vi "Certi Recall.vi"(4 "Value":string[][](array[string]), 5 "큐 입력":refnum<queue>, 6 "NumRows":u32, 7 "입력 클러스터":T1, 8 "에러 입력":errorcluster caption="에러 입력(에러 없음)", 10 "Text in":string, 11 "Func_ext in":string) -> (0 "에러 출력":errorcluster, 3 "Func_ext Out":string)   [LabVIEW 2020]
uses:
  Controls/Clst_Initialize Input.ctl
  Controls/Cmd_Var Data IO.ctl
  Variables/Global_Cal Info.vi
  Public/Polymorph/Table Initialize_Str.vi
  Public/Polymorph/Table Initialize_2D.vi
  Public/Polymorph/Rmv Empt Arr_2D Str.vi
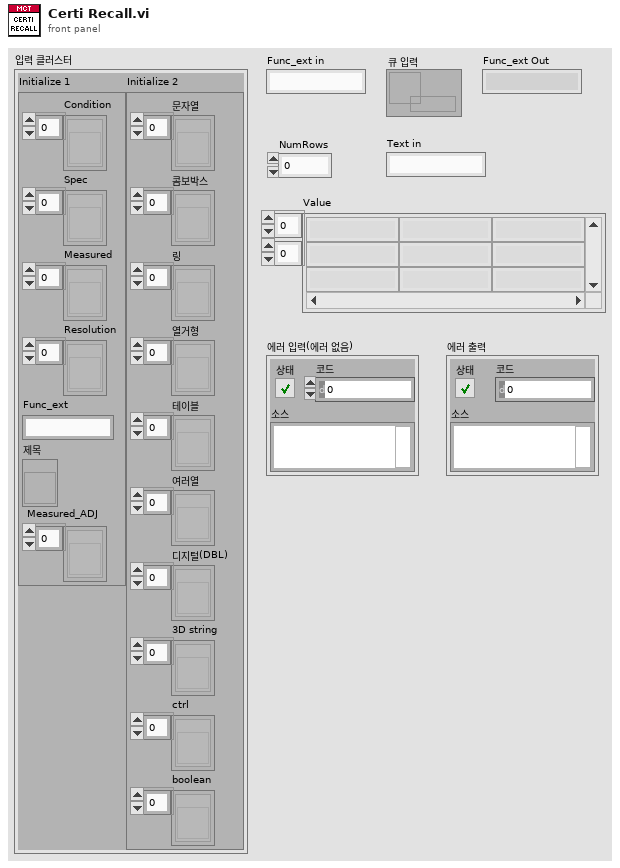
[diagram p1: front panel]
types:
  T1 = typedef "Clst_Initialize Input.ctl" = cluster{"Initialize 1":cluster{"Condition":refnum<vi>[], "Spec":refnum<vi>[], "Measured":refnum<vi>[], "Resolution":refnum<vi>[], "Func_ext":string, "제목":refnum<vi>, "Measured_ADJ":refnum<vi>[]}, "Initialize 2":cluster{"문자열":refnum<vi>[], "콤보박스":refnum<vi>[], "링":refnum<vi>[], "열거형":refnum<vi>[], "테이블":refnum<vi>[], "여러열":refnum<vi>[], "디지털(DBL)":refnum<vi>[], "3D string":refnum<vi>[], "ctrl":refnum<vi>[], "boolean":refnum<vi>[]}}
  T2 = cluster{"세부분류코드":string, "형식":string, "옵션":string, "측정기명":string, "EXCEL파일명":string, "TEMP":string}
  T3 = typedef "Cmd_Var Data IO.ctl" = enum16{"Condition", "Condition Default", "Condition_Temp", "Resolution", "Resolution Default", "Resolution Old", "Spec", "Spec Default", "Spec Old", "Spec Temp", "Result", "Result2", "Result3", "Result_Temp", "Result_ADJ", "Result_ADJ2", "STD1", "STD2", "STD3", "STD4", "STD5", "STD Temp", "CMC", "CMC Default"}
  T4 = enum8{"1단", "2단", "3단", "4단", "5단", "6단", "7단", "8단", "9단", "10단"}
  T5 = cluster{"교정 방향":string, "최대 용량":dbl, "최소눈금":dbl, "지시형태":string, "단위":string, "측정점 수":u8, "사용 기준기":string, "사용 기준기 2":string, "단 선택":enum8{"1단", "2단", "3단", "4단", "5단", "6단", "7단", "8단", "9단", "10단"}, "ItemNames":string[][]}
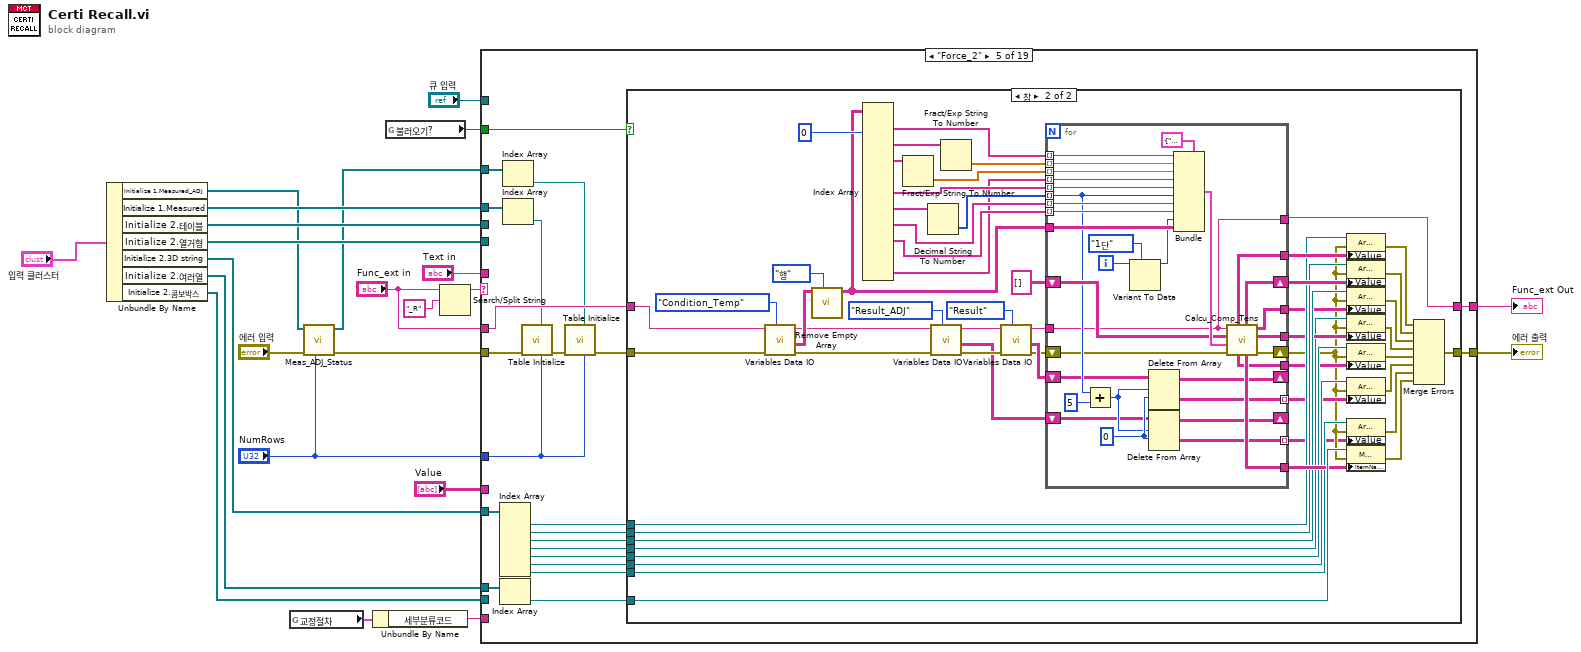
[diagram p0: block diagram]
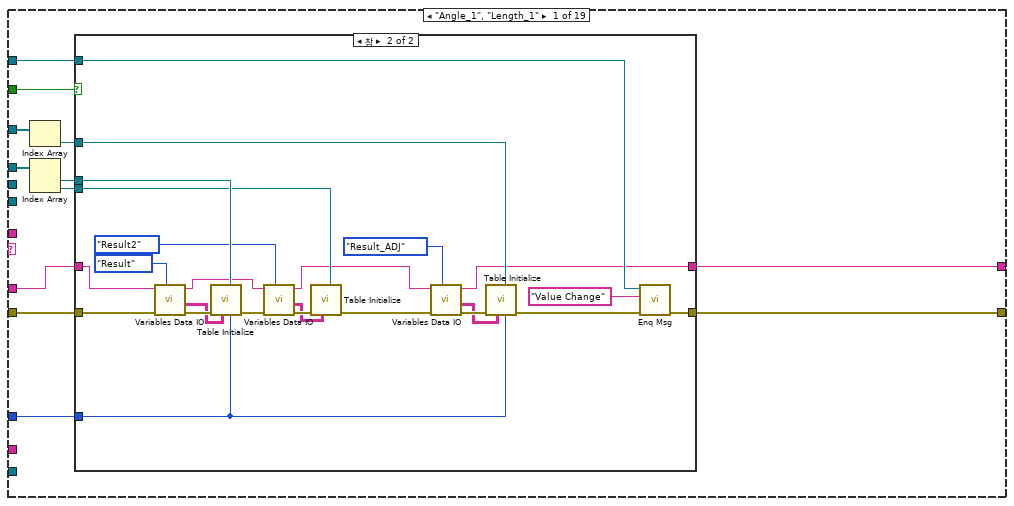
[diagram p2: hidden frame]
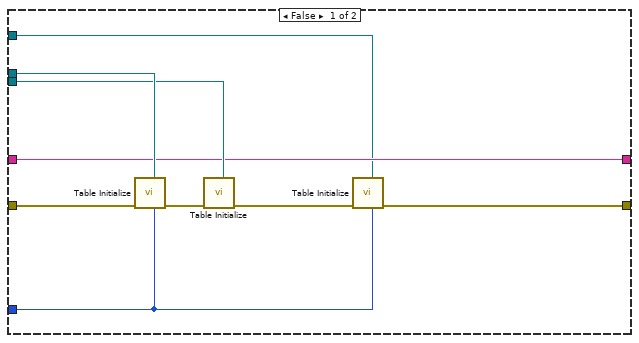
[diagram p3: hidden frame]
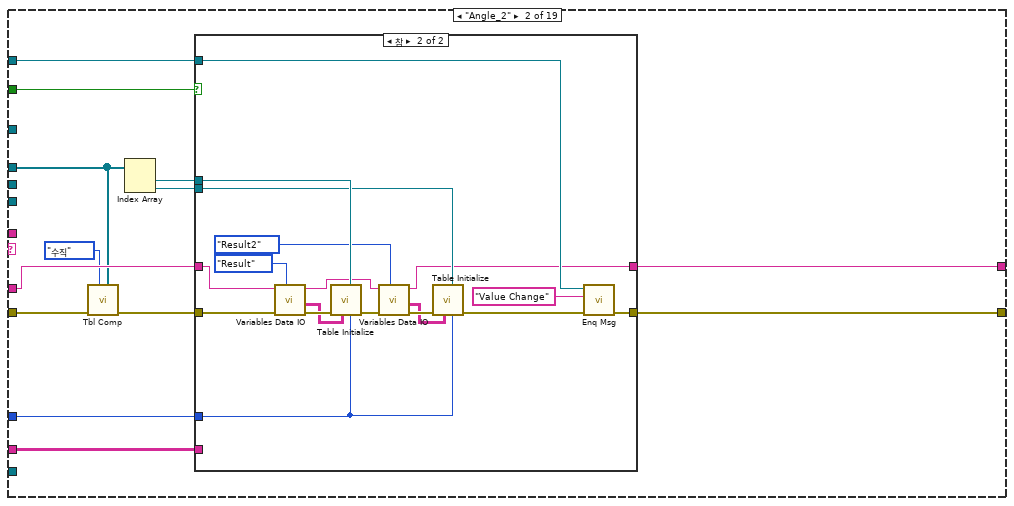
[diagram p4: hidden frame]
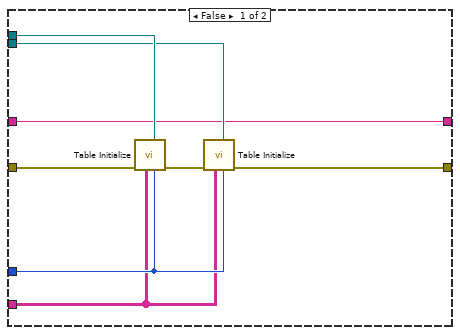
[diagram p5: hidden frame]
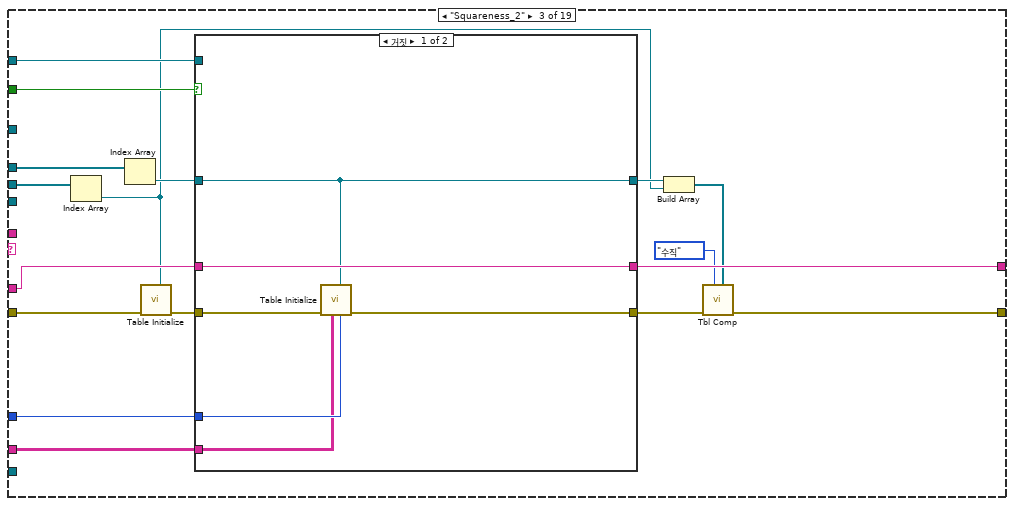
[diagram p6: hidden frame]
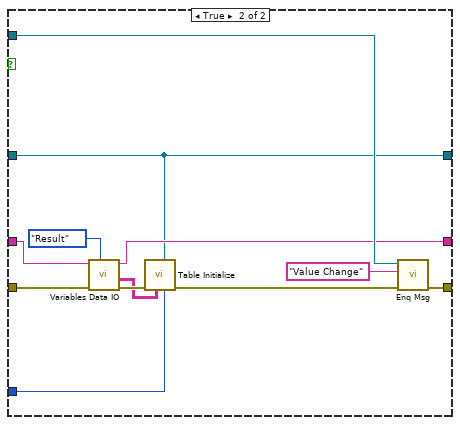
[diagram p7: hidden frame]
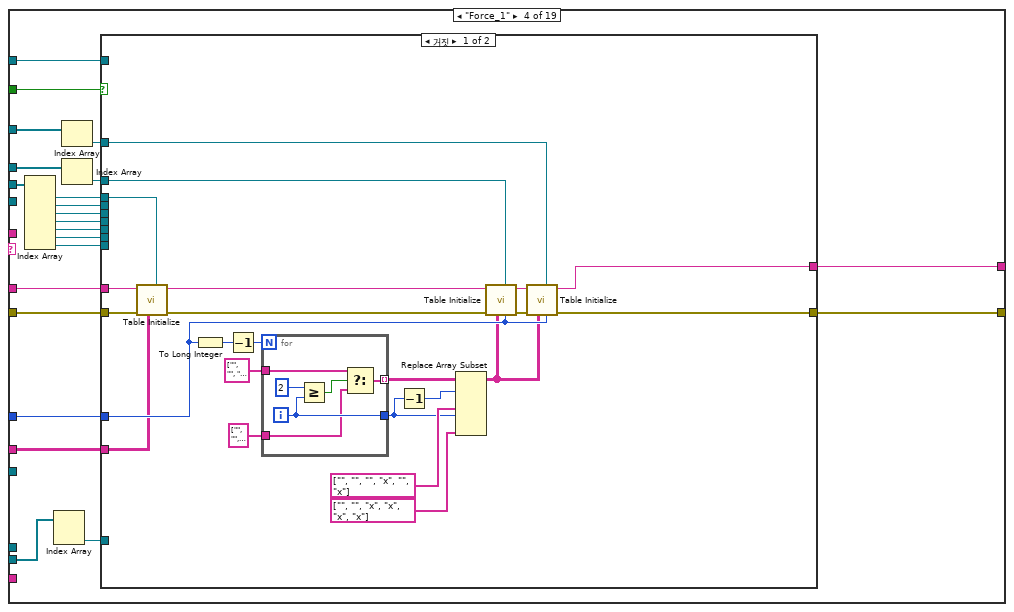
[diagram p8: hidden frame]
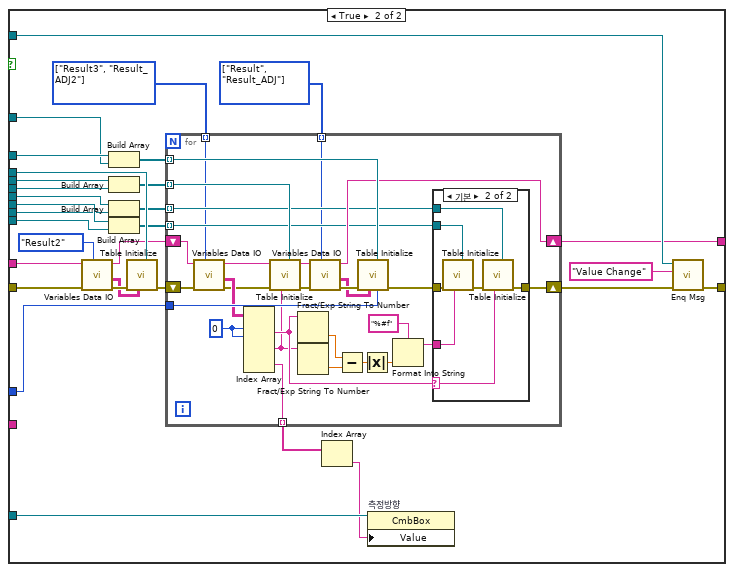
[diagram p9: hidden frame]
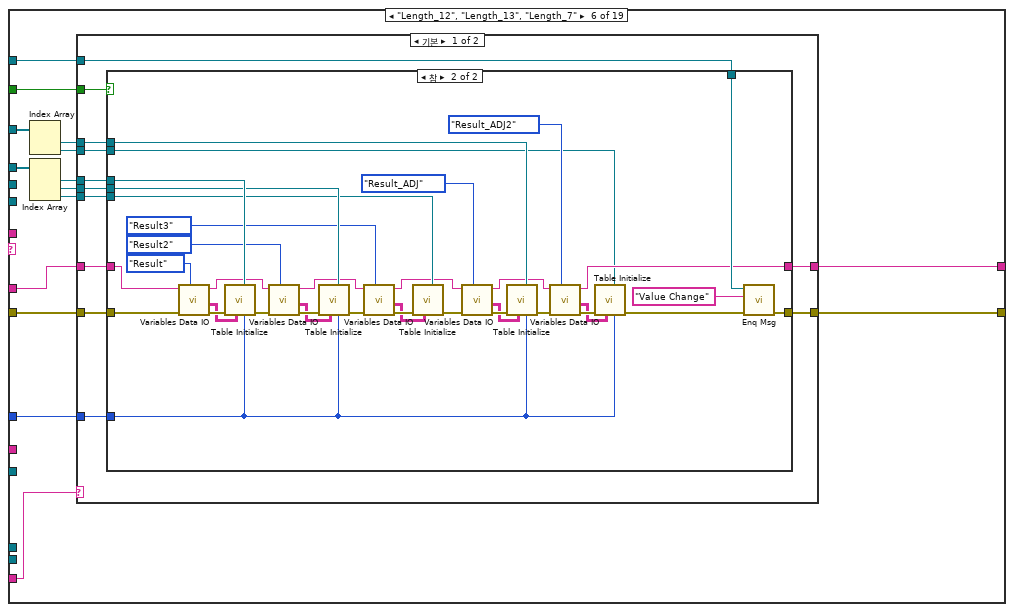
[diagram p12: hidden frame]
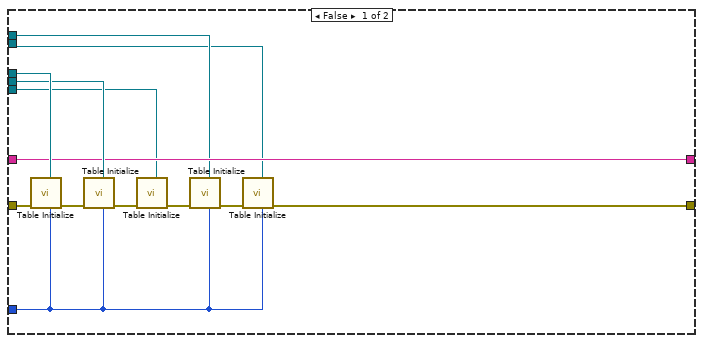
[diagram p13: hidden frame]
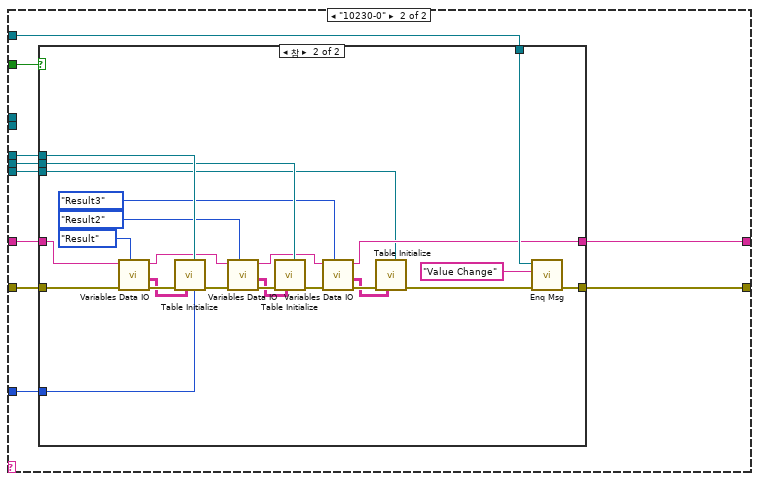
[diagram p14: hidden frame]
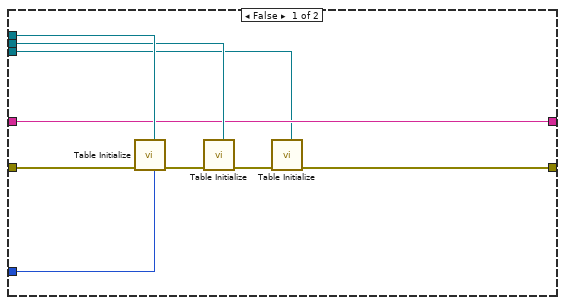
[diagram p15: hidden frame]
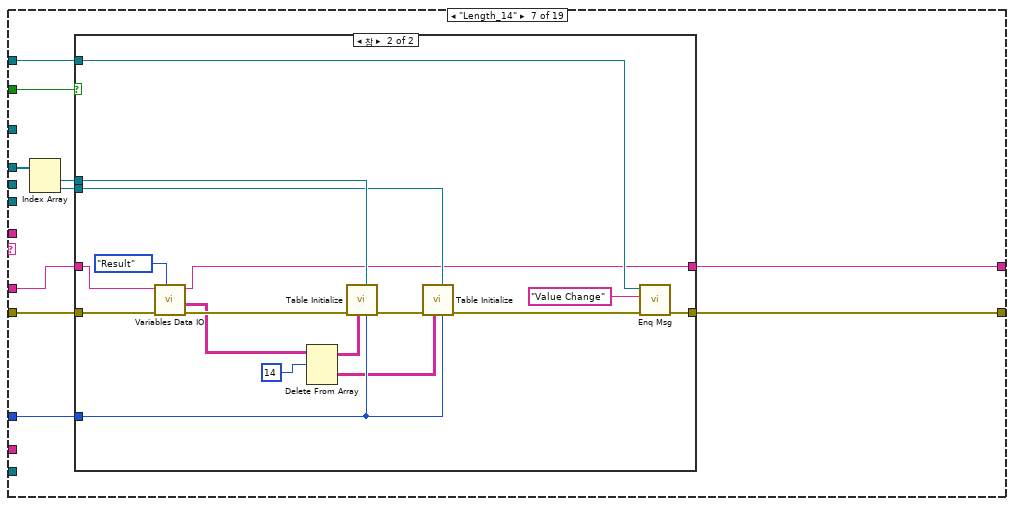
[diagram p16: hidden frame]
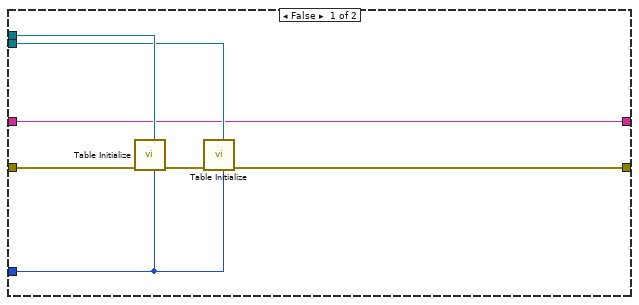
[diagram p17: hidden frame]
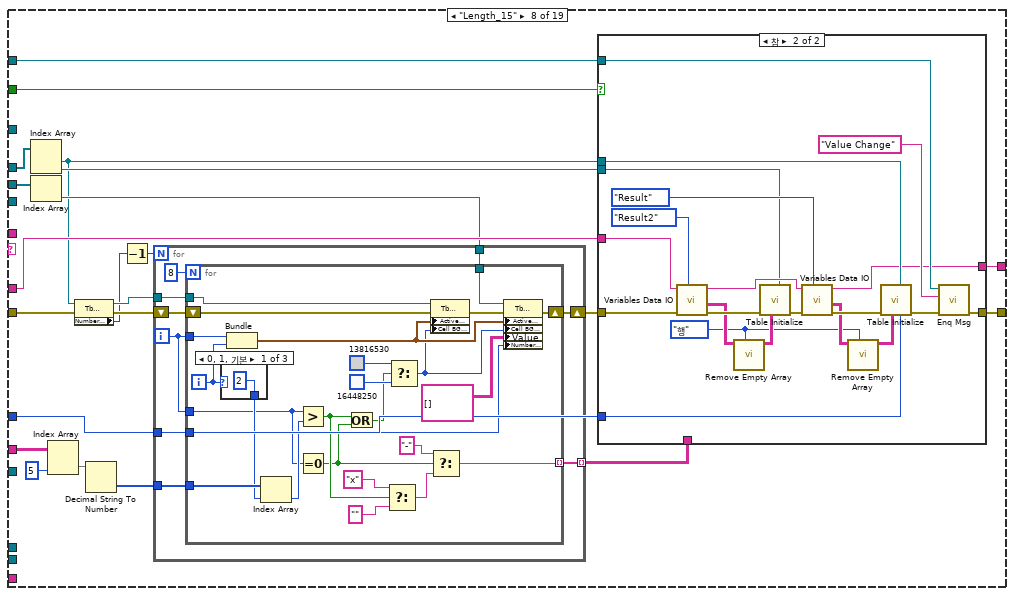
[diagram p18: hidden frame]
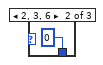
[diagram p19: hidden frame]
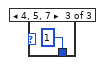
[diagram p20: hidden frame]
diagram:
  n1 = Unbundle By Name("입력 클러스터") -> ("Initialize 1.Measured_ADJ"=w1:refnum<vi>[], "Initialize 1.Measured"=w17:refnum<vi>[], "Initialize 2.테이블"=w20:refnum<vi>[], "Initialize 2.열거형"=w12:refnum<vi>[], "Initialize 2.3D string"=w18:refnum<vi>[], "Initialize 2.여러열"=w15:refnum<vi>[], "Initialize 2.콤보박스"=w16:refnum<vi>[])
  n2 = global read "Global_Cal Info.vi" "교정절차"() -> (w8:T2)
  n3 = call "Meas_ADJ_Status.vi"("NumRows"="NumRows", "에러 입력(에러 없음)"="에러 입력", "Measured_ADJ in"=w1) -> ("에러 출력"=w3:errorcluster, "Measured_ADJ out"=w5:refnum<vi>[])  [unwired: 7 in]
  n4 = Unbundle By Name(w8) -> ("세부분류코드"=w7:string)
  n5 = global read "Global_Cal Info.vi" "불러오기?"() -> (w22:bool)
  n6 = Search/Split String(string="Func_ext in", search string/char (-)="_R" ("검색 문자열/문자 (-)")) -> (substring before match=w10:string)  [unwired: 1 in, 2 out]
  n7 = case shown="\"Force_2\"" w10 {
    tunnel: "큐 입력" -> [w32 w79 w123 w163 _ w383 w496 w545 w618 w664 w711 w752 w884 w917 w968 w1015 w1063 w1137 w1171]
    tunnel: "NumRows" -> [w29 w78 w122 w162 w260 w381 w493 w524 w616 w661 w712 w749 w881 w914 w962 w1009 w1054 w1136 w1170]
    tunnel: [w30 w70 w112 w164 w279 w377 w494 w544 w614 w662 w710 w750 w882 w915 w959 w1006 w1052 w1135 w1169] -> w6
    tunnel: w22 -> [w28 w77 w121 w151 w278 w380 w492 w543 w615 w660 w713 w748 w880 w913 w964 w1011 w1062 w1134 w1168]
    tunnel: w3 -> [w31 w72 w115 w161 w262 w382 w495 w535 w617 w663 w714 w751 w883 w916 w963 w1010 w1059 w1133 w1167]
    tunnel: w17 -> [w33 w69 w117 w157 w264 w376 w497 w539 w619 w665 w707 w753 w885 w918 w967 w1014 w1050 w1132 w1166]
    tunnel: w20 -> [_ _ w116 w155 _ _ _ w540 _ _ _ w745 _ w912 _ _ _ _ _]
    tunnel: w16 -> [_ _ _ w154 _ _ _ _ _ _ w708 _ _ _ _ _ _ _ _]
    tunnel: "Value" -> [_ w74 w118 w152 _ _ _ w527 _ _ _ _ _ _ w961 w1008 _ _ _]
    tunnel: w15 -> [_ _ _ _ w277 _ _ _ _ _ _ _ _ _ _ _ _ _ _]
    tunnel: w18 -> [_ _ _ _ w275 _ _ _ _ _ _ _ _ _ _ _ _ _ _]
    tunnel: [w27 w76 w120 w150 w268 w379 w491 w542 w613 w659 w709 w747 w879 w910 w960 w1007 w1053 w1130 w1164] -> w14
    tunnel: "Text in" -> [_ _ _ _ _ _ _ _ _ _ _ _ _ _ w958 _ _ _ _]
    tunnel: w12 -> [_ _ _ _ _ _ _ _ _ _ _ _ _ _ _ _ w1061 _ _]
    tunnel: "Func_ext in" -> [w26 w75 w119 w149 w267 w378 w490 w541 w612 w658 w705 w746 w878 w909 w956 w1005 w1051 w1129 w1163]
    tunnel: w7 -> [_ _ _ _ _ w374 _ _ _ w654 _ w743 _ _ _ _ _ _ _]
    tunnel: w5 -> [w25 _ _ w148 w265 w373 _ _ _ w657 _ _ _ w908 w955 w1004 w1047 w1128 _]
    frame "Angle_1", "Length_1" {
      n8 = Index Array(array=w25) -> (element=w24:refnum<vi>)  [unwired: 1 in]
      n9 = Index Array(array=w33) -> (element #1=w34:refnum<vi>, element #2=w35:refnum<vi>)  [unwired: 2 in]
      n10 = case shown="참" w28 {
        tunnel: [w38 w64] -> w30
        tunnel: w26 -> [w40 w67]
        tunnel: w34 -> [w43 w61]
        tunnel: w29 -> [w37 w52]
        tunnel: w32 -> [_ w63]
        tunnel: w31 -> [w44 w62]
        tunnel: w35 -> [w41 w57]
        tunnel: [w40 w50] -> w27
        tunnel: w24 -> [w36 w53]
        frame False {
          n11 = call-poly "Table Initialize.vi"("행의 개수"=w37, "Table Ref"=w43, "에러 입력"=w44) -> ("에러 출력"=w42:errorcluster)  [unwired: 6 in, 2 out]
          n12 = call-poly "Table Initialize.vi"("Table Ref"=w41, "에러 입력"=w42) -> ("에러 출력"=w39:errorcluster)  [unwired: 7 in, 2 out]
          n13 = call-poly "Table Initialize.vi"("행의 개수"=w37, "Table Ref"=w36, "에러 입력"=w39) -> ("에러 출력"=w38:errorcluster)  [unwired: 6 in, 2 out]
        }
        frame True {
          n14 = call "Variables Data IO.vi"("Select"=Cmd_Var_Data_IO."Result", "error in"=w62, "Func_ext"=w67) -> ("error out"=w66:errorcluster, "Data Out"=w45:string[][], "Func_ext Out"=w56:string)  [unwired: 6 in]
          n15 = call-poly "Table Initialize.vi"("행의 개수"=w52, "Table Ref"=w61, "Value"=w45, "에러 입력"=w66) -> ("에러 출력"=w58:errorcluster)  [unwired: 5 in, 2 out]
          n16 = call "Variables Data IO.vi"("Select"=Cmd_Var_Data_IO."Result2", "error in"=w58, "Func_ext"=w56) -> ("error out"=w60:errorcluster, "Data Out"=w47:string[][], "Func_ext Out"=w51:string)  [unwired: 6 in]
          n17 = call-poly "Table Initialize.vi"("Table Ref"=w57, "Value"=w47, "에러 입력"=w60) -> ("에러 출력"=w55:errorcluster)  [unwired: 6 in, 2 out]
          n18 = call "Variables Data IO.vi"("Select"=Cmd_Var_Data_IO."Result_ADJ", "error in"=w55, "Func_ext"=w51) -> ("error out"=w49:errorcluster, "Data Out"=w46:string[][], "Func_ext Out"=w50:string)  [unwired: 6 in]
          n19 = call-poly "Table Initialize.vi"("행의 개수"=w52, "Table Ref"=w53, "Value"=w46, "에러 입력"=w49) -> ("에러 출력"=w54:errorcluster)  [unwired: 5 in, 2 out]
          n20 = call "Enq Msg.vi"("에러 입력(에러 없음)"=w54, "메세지"="Value Change", "큐 입력"=w63) -> ("에러 출력"=w64:errorcluster)  [unwired: 7 in, 1 out]
        }
      }
    }
    frame "Angle_2" {
      n21 = call "Tbl Comp.vi"("배열"=w69, "방향"=enum16{"수직", "수평"}."수직", "에러 입력"=w72) -> ("에러 출력"=w71:errorcluster)  [unwired: 6 in, 2 out]
      n22 = Index Array(array=w69) -> (element #1=w80:refnum<vi>, element #2=w81:refnum<vi>)  [unwired: 2 in]
      n23 = case shown="참" w77 {
        tunnel: [w85 w103] -> w70
        tunnel: w75 -> [w84 w106]
        tunnel: w80 -> [w88 w100]
        tunnel: w78 -> [w83 w92]
        tunnel: w79 -> [_ w102]
        tunnel: w71 -> [w89 w101]
        tunnel: w81 -> [w86 w95]
        tunnel: [w84 w93] -> w76
        tunnel: w74 -> [w82 _]
        frame False {
          n24 = call-poly "Table Initialize.vi"("행의 개수"=w83, "Table Ref"=w88, "Value"=w82, "에러 입력"=w89) -> ("에러 출력"=w87:errorcluster)  [unwired: 5 in, 2 out]
          n25 = call-poly "Table Initialize.vi"("행의 개수"=w83, "Table Ref"=w86, "Value"=w82, "에러 입력"=w87) -> ("에러 출력"=w85:errorcluster)  [unwired: 5 in, 2 out]
        }
        frame True {
          n26 = call "Variables Data IO.vi"("Select"=Cmd_Var_Data_IO."Result", "error in"=w101, "Func_ext"=w106) -> ("error out"=w105:errorcluster, "Data Out"=w90:string[][], "Func_ext Out"=w94:string)  [unwired: 6 in]
          n27 = call-poly "Table Initialize.vi"("행의 개수"=w92, "Table Ref"=w100, "Value"=w90, "에러 입력"=w105) -> ("에러 출력"=w97:errorcluster)  [unwired: 5 in, 2 out]
          n28 = call "Variables Data IO.vi"("Select"=Cmd_Var_Data_IO."Result2", "error in"=w97, "Func_ext"=w94) -> ("error out"=w99:errorcluster, "Data Out"=w91:string[][], "Func_ext Out"=w93:string)  [unwired: 6 in]
          n29 = call-poly "Table Initialize.vi"("행의 개수"=w92, "Table Ref"=w95, "Value"=w91, "에러 입력"=w99) -> ("에러 출력"=w96:errorcluster)  [unwired: 5 in, 2 out]
          n30 = call "Enq Msg.vi"("에러 입력(에러 없음)"=w96, "메세지"="Value Change", "큐 입력"=w102) -> ("에러 출력"=w103:errorcluster)  [unwired: 7 in, 1 out]
        }
      }
    }
    frame "Squareness_2" {
      n31 = Index Array(array=w116) -> (element=w109:refnum<vi>)  [unwired: 1 in]
      n32 = Index Array(array=w117) -> (element=w124:refnum<vi>)  [unwired: 1 in]
      n33 = call-poly "Table Initialize.vi"("Table Ref"=w109, "에러 입력"=w115) -> ("에러 출력"=w114:errorcluster)  [unwired: 7 in, 2 out]
      n34 = case shown="거짓" w121 {
        tunnel: [w129 w138] -> w113
        tunnel: w119 -> [w128 w141]
        tunnel: w124 -> [w125 w131]
        tunnel: w122 -> [w127 w134]
        tunnel: w123 -> [_ w137]
        tunnel: w114 -> [w130 w136]
        tunnel: [w128 w135] -> w120
        tunnel: w118 -> [w126 _]
        tunnel: [w125 w131] -> w110
        frame False {
          n35 = call-poly "Table Initialize.vi"("행의 개수"=w127, "Table Ref"=w125, "Value"=w126, "에러 입력"=w130) -> ("에러 출력"=w129:errorcluster)  [unwired: 5 in, 2 out]
        }
        frame True {
          n36 = call "Variables Data IO.vi"("Select"=Cmd_Var_Data_IO."Result", "error in"=w136, "Func_ext"=w141) -> ("error out"=w140:errorcluster, "Data Out"=w133:string[][], "Func_ext Out"=w135:string)  [unwired: 6 in]
          n37 = call-poly "Table Initialize.vi"("행의 개수"=w134, "Table Ref"=w131, "Value"=w133, "에러 입력"=w140) -> ("에러 출력"=w132:errorcluster)  [unwired: 5 in, 2 out]
          n38 = call "Enq Msg.vi"("에러 입력(에러 없음)"=w132, "메세지"="Value Change", "큐 입력"=w137) -> ("에러 출력"=w138:errorcluster)  [unwired: 7 in, 1 out]
        }
      }
      n39 = Build Array(w110, w109) -> (w108:refnum<vi>[])
      n40 = call "Tbl Comp.vi"("배열"=w108, "방향"=enum16{"수직", "수평"}."수직", "에러 입력"=w113) -> ("에러 출력"=w112:errorcluster)  [unwired: 6 in, 2 out]
    }
    frame "Force_1" {
      n41 = Index Array(array=w155) -> (element #1=w160:refnum<vi>, element #2=w159:refnum<vi>, element #3=w143:refnum<vi>, element #4=w158:refnum<vi>, element #5=w146:refnum<vi>, element #6=w145:refnum<vi>, element #7=w144:refnum<vi>)  [unwired: 7 in]
      n42 = Index Array(array=w154) -> (element #2=w153:refnum<vi>)  [unwired: 2 in, 1 out]
      n43 = Index Array(array=w148) -> (element=w147:refnum<vi>)  [unwired: 1 in]
      n44 = Index Array(array=w157) -> (element=w156:refnum<vi>)  [unwired: 1 in]
      n45 = case shown="거짓" w151 {
        tunnel: [w170 w221] -> w164
        tunnel: w149 -> [w172 w206]
        tunnel: w156 -> [w184 w200]
        tunnel: w162 -> [w168 w220]
        tunnel: w163 -> [_ w219]
        tunnel: w161 -> [w173 w207]
        tunnel: w160 -> [w183 w216]
        tunnel: w159 -> [_ w213]
        tunnel: w158 -> [_ w212]
        tunnel: w153 -> [_ w215]
        tunnel: w152 -> [w165 _]
        tunnel: [w172 w214] -> w150
        tunnel: w147 -> [w169 w199]
        tunnel: w146 -> [_ w211]
        tunnel: w145 -> [_ w196]
        tunnel: w144 -> [_ w195]
        tunnel: w143 -> [_ w193]
        frame False {
          n46 = call-poly "Table Initialize.vi"("Table Ref"=w183, "Value"=w165, "에러 입력"=w173) -> ("에러 출력"=w167:errorcluster)  [unwired: 6 in, 2 out]
          n47 = To Long Integer(number=w168) -> (32bit integer=w181:i32)
          n48 = Decrement(x=w181) -> (x-1=w182:i32)
          n49 = for {
            N: w182 -> [_]
            tunnel: [w187] -> w174 mode=indexing
            tunnel: [w190] -> w176
            tunnel: string[] ["", "", "", "", "", ""] -> [w189]
            tunnel: string[] ["", "", "", "ⅹ", "ⅹ", "ⅹ"] -> [w188]
            i -> [w190]
            n50 = Greater Or Equal?(x=2, y=w190) -> (x >= y?=w186:bool)
            n51 = Select(t=w188, s=w186, f=w189) -> (s? t:f=w187:string[])
          }
          n52 = Decrement(x=w176) -> (x-1=w177:i32)
          n53 = Replace Array Subset(array=w174, new element #1=string[] ["", "", "", "ⅹ", "", "ⅹ"], index (row) #1=w177, new element #2=string[] ["", "", "ⅹ", "ⅹ", "ⅹ", "ⅹ"], index (row) #2=w176) -> (w166:string[][])  [unwired: 2 in]
          n54 = call-poly "Table Initialize.vi"("행의 개수"=w168, "Table Ref"=w184, "Value"=w166, "에러 입력"=w167) -> ("에러 출력"=w171:errorcluster)  [unwired: 5 in, 2 out]
          n55 = call-poly "Table Initialize.vi"("행의 개수"=w168, "Table Ref"=w169, "Value"=w166, "에러 입력"=w171) -> ("에러 출력"=w170:errorcluster)  [unwired: 5 in, 2 out]
        }
        frame True {
          w202 = T3[] [enum."Result3", enum."Result_ADJ2"] items=["Condition", "Condition Default", "Condition_Temp", "Resolution", "Resolution Default", "Resolution Old", "Spec", "Spec Default", "Spec Old", "Spec Temp", "Result", "Result2", "Result3", "Result_Temp", "Result_ADJ", "Result_ADJ2", "STD1", "STD2", "STD3", "STD4", "STD5", "STD Temp", "CMC", "CMC Default"]
          w203 = T3[] [enum."Result", enum."Result_ADJ"] items=["Condition", "Condition Default", "Condition_Temp", "Resolution", "Resolution Default", "Resolution Old", "Spec", "Spec Default", "Spec Old", "Spec Temp", "Result", "Result2", "Result3", "Result_Temp", "Result_ADJ", "Result_ADJ2", "STD1", "STD2", "STD3", "STD4", "STD5", "STD Temp", "CMC", "CMC Default"]
          n56 = call "Variables Data IO.vi"("Select"=Cmd_Var_Data_IO."Result2", "error in"=w207, "Func_ext"=w206) -> ("error out"=w208:errorcluster, "Data Out"=w191:string[][], "Func_ext Out"=w205:string)  [unwired: 6 in]
          n57 = Build Array(w200, w199) -> (w201:refnum<vi>[])
          n58 = Build Array(w213, w193) -> (w194:refnum<vi>[])
          n59 = Build Array(w212, w196) -> (w198:refnum<vi>[])
          n60 = Build Array(w211, w195) -> (w197:refnum<vi>[])
          n61 = call-poly "Table Initialize.vi"("Table Ref"=w216, "Value"=w191, "에러 입력"=w208) -> ("에러 출력"=w204:errorcluster)  [unwired: 6 in, 2 out]
          n62 = for {
            tunnel: w220 -> [w249]
            tunnel: w201 -> [w247] mode=indexing
            tunnel: w194 -> [w245] mode=indexing
            tunnel: w198 -> [w243] mode=indexing
            tunnel: w197 -> [w242] mode=indexing
            tunnel: [w238] -> w210 mode=indexing
            shift-right: [w246] -> w214
            shift-left: w205 -> [w232]
            shift-right: [w224] -> w217
            shift-left: w204 -> [w230]
            tunnel: w203 -> [w229] mode=indexing
            tunnel: w202 -> [w228] mode=indexing
            w241 = 0 ("인덱스 (행)")
            n63 = call "Variables Data IO.vi"("Select"=w228, "error in"=w230, "Func_ext"=w232) -> ("error out"=w227:errorcluster, "Data Out"=w244:string[][], "Func_ext Out"=w231:string)  [unwired: 6 in]
            n64 = Index Array(array=w244, index (row) #1=w241, index (col) #1=w241) -> (element #1=w240:string, element #2=w239:string, element #3=w238:string)  [unwired: 4 in]
            n65 = Fract/Exp String To Number(string=w240) -> (number=w234:dbl)  [unwired: 3 in, 1 out]
            n66 = Fract/Exp String To Number(string=w239) -> (number=w233:dbl)  [unwired: 3 in, 1 out]
            n67 = call "Variables Data IO.vi"("Select"=w229, "error in"=w227, "Func_ext"=w231) -> ("error out"=w248:errorcluster, "Data Out"=w223:string[][], "Func_ext Out"=w246:string)  [unwired: 6 in]
            n68 = Subtract(x=w234, y=w233) -> (x-y=w235:dbl)
            n69 = call-poly "Table Initialize.vi"("행의 개수"=w249, "Table Ref"=w247, "Value"=w223, "에러 입력"=w248) -> ("에러 출력"=w226:errorcluster)  [unwired: 5 in, 2 out]
            n70 = call-poly "Table Initialize.vi"("Table Ref"=w245, "Value"=w239, "에러 입력"=w226) -> ("에러 출력"=w225:errorcluster)  [unwired: 6 in, 2 out]
            n71 = Absolute Value(x=w235) -> (abs(x)=w237:dbl)
            n72 = Format Into String(format string="%#f" ("포맷 문자열"), w237) -> (resulting string=w222:string)  [unwired: 2 in, 1 out]
            n73 = case shown="기본" w240 {
              selector: w240 -> [_ w251]
              tunnel: [w250 w254] -> w224
              tunnel: w243 -> [_ w257]
              tunnel: w225 -> [w250 w256]
              tunnel: w242 -> [_ w253]
              tunnel: w222 -> [_ w252]
              frame "ⅹ" {
              }
              frame Default {
                n74 = call-poly "Table Initialize.vi"("Table Ref"=w257, "Value"=w251, "에러 입력"=w256) -> ("에러 출력"=w255:errorcluster)  [unwired: 6 in, 2 out]
                n75 = call-poly "Table Initialize.vi"("Table Ref"=w253, "Value"=w252, "에러 입력"=w255) -> ("에러 출력"=w254:errorcluster)  [unwired: 6 in, 2 out]
              }
            }
          }
          n76 = Index Array(array=w210) -> (element=w192:string)  [unwired: 1 in]
          n77 = property on="측정방향" class="CmbBox"(reference=w215, "Value"=w192) -> ()  [unwired: 1 in, 2 out]
          n78 = call "Enq Msg.vi"("에러 입력(에러 없음)"=w217, "메세지"="Value Change", "큐 입력"=w219) -> ("에러 출력"=w221:errorcluster)  [unwired: 7 in, 1 out]
        }
      }
    }
    frame "Force_2" {
      n79 = Index Array(array=w275) -> (element #1=w274:refnum<vi>, element #2=w273:refnum<vi>, element #3=w272:refnum<vi>, element #4=w271:refnum<vi>, element #5=w269:refnum<vi>, element #6=w270:refnum<vi>, element #7=w266:refnum<vi>)  [unwired: 7 in]
      n80 = Index Array(array=w277) -> (element=w276:refnum<vi>)  [unwired: 1 in]
      n81 = Index Array(array=w265) -> (element=w258:refnum<vi>)  [unwired: 1 in]
      n82 = Index Array(array=w264) -> (element=w259:refnum<vi>)  [unwired: 1 in]
      n83 = call-poly "Table Initialize.vi"("행의 개수"=w260, "Table Ref"=w259, "에러 입력"=w262) -> ("에러 출력"=w263:errorcluster)  [unwired: 6 in, 2 out]
      n84 = call-poly "Table Initialize.vi"("행의 개수"=w260, "Table Ref"=w258, "에러 입력"=w263) -> ("에러 출력"=w261:errorcluster)  [unwired: 6 in, 2 out]
      n85 = case shown="참" w278 {
        tunnel: [w280 w318] -> w279
        tunnel: w267 -> [w281 w284]
        tunnel: w261 -> [w280 w282]
        tunnel: w274 -> [_ w330]
        tunnel: w276 -> [_ w335]
        tunnel: w273 -> [_ w329]
        tunnel: w271 -> [_ w326]
        tunnel: w272 -> [_ w331]
        tunnel: w269 -> [_ w325]
        tunnel: w270 -> [_ w317]
        tunnel: [w281 w298] -> w268
        tunnel: w266 -> [_ w295]
        frame False {
        }
        frame True {
          n86 = call "Variables Data IO.vi"("Select"=Cmd_Var_Data_IO."Condition_Temp", "error in"=w282, "Func_ext"=w284) -> ("error out"=w283:errorcluster, "Data Out"=w303:string[][], "Func_ext Out"=w286:string)  [unwired: 6 in]
          n87 = call-poly "Remove Empty Array.vi"("조건"=enum16{"행", "열", "행,열"}."행", "Data in"=w303) -> ("Data out"=w302:string[][])  [unwired: 8 in, 1 out]
          n88 = Index Array(array=w302, index (col) #1=0 ("비활성화된 인덱스 (열)")) -> (element #1=w315:string[], element #2=w314:string[], element #3=w312:string[], element #5=w310:string[], element #6=w309:string[], element #7=w307:string[], element #8=w306:string[], element #10=w305:string[])  [unwired: 19 in, 2 out]
          n89 = Fract/Exp String To Number(string=w312) -> (number=w311:dbl[])  [unwired: 3 in, 1 out]
          n90 = Decimal String To Number(string=w309) -> (number=w308:i32[])  [unwired: 2 in, 1 out]
          n91 = call "Variables Data IO.vi"("Select"=Cmd_Var_Data_IO."Result_ADJ", "error in"=w283, "Func_ext"=w286) -> ("error out"=w291:errorcluster, "Data Out"=w288:string[][], "Func_ext Out"=w290:string)  [unwired: 6 in]
          n92 = Fract/Exp String To Number(string=w314) -> (number=w313:dbl[])  [unwired: 3 in, 1 out]
          n93 = call "Variables Data IO.vi"("Select"=Cmd_Var_Data_IO."Result", "error in"=w291, "Func_ext"=w290) -> ("error out"=w287:errorcluster, "Data Out"=w289:string[][], "Func_ext Out"=w285:string)  [unwired: 6 in]
          n94 = for {
            tunnel: w302 -> [w368]
            tunnel: [w367] -> w334
            tunnel: [w365] -> w332
            tunnel: [w364] -> w328
            tunnel: [w363] -> w327
            tunnel: [w362] -> w324
            shift-right: [w361] -> w294
            shift-left: w287 -> [w338]
            tunnel: w315 -> [w360] mode=indexing
            tunnel: w313 -> [w359] mode=indexing
            tunnel: w311 -> [w358] mode=indexing
            tunnel: w305 -> [w357] mode=indexing
            tunnel: w310 -> [w356] mode=indexing
            tunnel: w308 -> [w350] mode=indexing
            tunnel: w307 -> [w355] mode=indexing
            tunnel: w306 -> [w354] mode=indexing
            shift-right: [w366] -> w333
            shift-left: string[][][] [] ("condition out") -> [w353]
            shift-right: [w348] -> _
            shift-left: w289 -> [w349]
            tunnel: [w347] -> w300 mode=indexing
            tunnel: [w339] -> w298
            shift-right: [w341] -> _
            shift-left: w288 -> [w342]
            tunnel: [w340] -> w293 mode=indexing
            tunnel: w285 -> [w339]
            i -> [w352]
            w344 = 0 ("인덱스 (행)")
            n95 = Add(x=w350, y=5) -> (x+y=w343:i32)
            n96 = Variant To Data(type=T4."1단" ("단 선택"), Variant=w352) -> (data=w351:T4)  [unwired: 1 in, 1 out]
            n97 = Delete From Array(array=w349, length=w343, index (row)=w344) -> (deleted portion=w347:string[][], array with subset deleted=w348:string[][])  [unwired: 1 in]
            n98 = Delete From Array(array=w342, length=w343, index (row)=w344) -> (deleted portion=w340:string[][], array with subset deleted=w341:string[][])  [unwired: 1 in]
            n99 = Bundle(cluster=T5 {"교정 방향"="", "최대 용량"=0.0, "최소눈금"=0.0, "지시형태"="", "단위"="", "측정점 수"=0, "사용 기준기"="", "사용 기준기 2"="", "단 선택"=enum."1단", "ItemNames"=[]} ("클러스터"), "교정 방향"=w360, "최대 용량"=w359, "최소눈금"=w358, "지시형태"=w357, "단위"=w356, "측정점 수"=w350, "사용 기준기"=w355, "사용 기준기 2"=w354, "단 선택"=w351, "ItemNames"=w368) -> (w369:T5)
            n100 = call "Calcu_Comp_Tens.vi"("error in"=w338, "클러스터"=w369, "Condition set"=w353, "Func_ext"=w339) -> ("error out"=w361:errorcluster, "Resolution"=w363:string[][][], "Spec Out"=w364:string[][][], "ItemNames 출력"=w367:string[][], "condition out"=w366:string[][][], "cmc out"=w362:string[][][], "Spec Default"=w365:string[][][])  [unwired: 1 out]
          }
          n101 = property class="Arr (엄격한)"(reference=w330, error in=w294, "Value"=w332) -> (error out=w323:errorcluster)  [unwired: 1 out]
          n102 = property class="Arr (엄격한)"(reference=w329, error in=w294, "Value"=w333) -> (error out=w322:errorcluster)  [unwired: 1 out]
          n103 = property class="Arr (엄격한)"(reference=w331, error in=w294, "Value"=w328) -> (error out=w299:errorcluster)  [unwired: 1 out]
          n104 = property class="Arr (엄격한)"(reference=w326, error in=w294, "Value"=w327) -> (error out=w321:errorcluster)  [unwired: 1 out]
          n105 = property class="Arr (엄격한)"(reference=w325, error in=w294, "Value"=w324) -> (error out=w320:errorcluster)  [unwired: 1 out]
          n106 = property class="Arr (엄격한)"(reference=w317, error in=w294, "Value"=w300) -> (error out=w319:errorcluster)  [unwired: 1 out]
          n107 = property class="Arr (엄격한)"(reference=w295, error in=w294, "Value"=w293) -> (error out=w296:errorcluster)  [unwired: 1 out]
          n108 = property class="MCListbox (엄격한)"(reference=w335, error in=w294, "ItemNames"=w334) -> (error out=w297:errorcluster)  [unwired: 1 out]
          n109 = Merge Errors(w323, w322, w299, w321, w320, w319, w296, w297) -> (w318:errorcluster)
        }
      }
    }
    frame "Length_12", "Length_13", "Length_7" {
      n110 = Index Array(array=w373) -> (element #1=w372:refnum<vi>, element #2=w371:refnum<vi>)  [unwired: 2 in]
      n111 = Index Array(array=w376) -> (element #1=w384:refnum<vi>, element #2=w385:refnum<vi>, element #3=w375:refnum<vi>)  [unwired: 3 in]
      n112 = case shown="기본" w374 {
        tunnel: w385 -> [w397 w456]
        tunnel: w384 -> [w396 w455]
        tunnel: w383 -> [w395 w454]
        tunnel: w382 -> [w394 w453]
        tunnel: w381 -> [w393 w452]
        tunnel: w380 -> [w392 w451]
        tunnel: [w391 w450] -> w379
        tunnel: w378 -> [w390 w449]
        tunnel: [w389 w448] -> w377
        tunnel: w375 -> [w388 w447]
        tunnel: w372 -> [w387 _]
        tunnel: w371 -> [w386 _]
        frame Default {
          n113 = case shown="참" w392 {
            tunnel: [w400 w442] -> w389
            tunnel: w390 -> [w406 w445]
            tunnel: w396 -> [w409 w439]
            tunnel: w393 -> [w399 w417]
            tunnel: w395 -> [_ w441]
            tunnel: w394 -> [w410 w440]
            tunnel: w397 -> [w407 w435]
            tunnel: [w406 w420] -> w391
            tunnel: w388 -> [w404 w430]
            tunnel: w387 -> [w402 w426]
            tunnel: w386 -> [w398 w418]
            frame False {
              n114 = call-poly "Table Initialize.vi"("행의 개수"=w399, "Table Ref"=w409, "에러 입력"=w410) -> ("에러 출력"=w408:errorcluster)  [unwired: 6 in, 2 out]
              n115 = call-poly "Table Initialize.vi"("행의 개수"=w399, "Table Ref"=w407, "에러 입력"=w408) -> ("에러 출력"=w405:errorcluster)  [unwired: 6 in, 2 out]
              n116 = call-poly "Table Initialize.vi"("Table Ref"=w404, "에러 입력"=w405) -> ("에러 출력"=w403:errorcluster)  [unwired: 7 in, 2 out]
              n117 = call-poly "Table Initialize.vi"("행의 개수"=w399, "Table Ref"=w402, "에러 입력"=w403) -> ("에러 출력"=w401:errorcluster)  [unwired: 6 in, 2 out]
              n118 = call-poly "Table Initialize.vi"("행의 개수"=w399, "Table Ref"=w398, "에러 입력"=w401) -> ("에러 출력"=w400:errorcluster)  [unwired: 6 in, 2 out]
            }
            frame True {
              n119 = call "Variables Data IO.vi"("Select"=Cmd_Var_Data_IO."Result", "error in"=w440, "Func_ext"=w445) -> ("error out"=w444:errorcluster, "Data Out"=w411:string[][], "Func_ext Out"=w434:string)  [unwired: 6 in]
              n120 = call-poly "Table Initialize.vi"("행의 개수"=w417, "Table Ref"=w439, "Value"=w411, "에러 입력"=w444) -> ("에러 출력"=w436:errorcluster)  [unwired: 5 in, 2 out]
              n121 = call "Variables Data IO.vi"("Select"=Cmd_Var_Data_IO."Result2", "error in"=w436, "Func_ext"=w434) -> ("error out"=w438:errorcluster, "Data Out"=w412:string[][], "Func_ext Out"=w432:string)  [unwired: 6 in]
              n122 = call-poly "Table Initialize.vi"("행의 개수"=w417, "Table Ref"=w435, "Value"=w412, "에러 입력"=w438) -> ("에러 출력"=w433:errorcluster)  [unwired: 5 in, 2 out]
              n123 = call "Variables Data IO.vi"("Select"=Cmd_Var_Data_IO."Result3", "error in"=w433, "Func_ext"=w432) -> ("error out"=w431:errorcluster, "Data Out"=w413:string[][], "Func_ext Out"=w425:string)  [unwired: 6 in]
              n124 = call-poly "Table Initialize.vi"("Table Ref"=w430, "Value"=w413, "에러 입력"=w431) -> ("에러 출력"=w428:errorcluster)  [unwired: 6 in, 2 out]
              n125 = call "Variables Data IO.vi"("Select"=Cmd_Var_Data_IO."Result_ADJ", "error in"=w428, "Func_ext"=w425) -> ("error out"=w424:errorcluster, "Data Out"=w414:string[][], "Func_ext Out"=w421:string)  [unwired: 6 in]
              n126 = call-poly "Table Initialize.vi"("행의 개수"=w417, "Table Ref"=w426, "Value"=w414, "에러 입력"=w424) -> ("에러 출력"=w423:errorcluster)  [unwired: 5 in, 2 out]
              n127 = call "Variables Data IO.vi"("Select"=Cmd_Var_Data_IO."Result_ADJ2", "error in"=w423, "Func_ext"=w421) -> ("error out"=w419:errorcluster, "Data Out"=w415:string[][], "Func_ext Out"=w420:string)  [unwired: 6 in]
              n128 = call-poly "Table Initialize.vi"("행의 개수"=w417, "Table Ref"=w418, "Value"=w415, "에러 입력"=w419) -> ("에러 출력"=w416:errorcluster)  [unwired: 5 in, 2 out]
              n129 = call "Enq Msg.vi"("에러 입력(에러 없음)"=w416, "메세지"="Value Change", "큐 입력"=w441) -> ("에러 출력"=w442:errorcluster)  [unwired: 7 in, 1 out]
            }
          }
        }
        frame "10230-0" {
          n130 = case shown="참" w451 {
            tunnel: [w458 w485] -> w448
            tunnel: w449 -> [w461 w488]
            tunnel: w455 -> [w464 w482]
            tunnel: w452 -> [w460 w476]
            tunnel: w454 -> [_ w484]
            tunnel: w453 -> [w465 w483]
            tunnel: w456 -> [w462 w478]
            tunnel: [w461 w473] -> w450
            tunnel: w447 -> [w457 w470]
            frame False {
              n131 = call-poly "Table Initialize.vi"("행의 개수"=w460, "Table Ref"=w464, "에러 입력"=w465) -> ("에러 출력"=w463:errorcluster)  [unwired: 6 in, 2 out]
              n132 = call-poly "Table Initialize.vi"("Table Ref"=w462, "에러 입력"=w463) -> ("에러 출력"=w459:errorcluster)  [unwired: 7 in, 2 out]
              n133 = call-poly "Table Initialize.vi"("Table Ref"=w457, "에러 입력"=w459) -> ("에러 출력"=w458:errorcluster)  [unwired: 7 in, 2 out]
            }
            frame True {
              n134 = call "Variables Data IO.vi"("Select"=Cmd_Var_Data_IO."Result", "error in"=w483, "Func_ext"=w488) -> ("error out"=w487:errorcluster, "Data Out"=w468:string[][], "Func_ext Out"=w477:string)  [unwired: 6 in]
              n135 = call-poly "Table Initialize.vi"("행의 개수"=w476, "Table Ref"=w482, "Value"=w468, "에러 입력"=w487) -> ("에러 출력"=w479:errorcluster)  [unwired: 5 in, 2 out]
              n136 = call "Variables Data IO.vi"("Select"=Cmd_Var_Data_IO."Result2", "error in"=w479, "Func_ext"=w477) -> ("error out"=w481:errorcluster, "Data Out"=w467:string[][], "Func_ext Out"=w474:string)  [unwired: 6 in]
              n137 = call-poly "Table Initialize.vi"("Table Ref"=w478, "Value"=w467, "에러 입력"=w481) -> ("에러 출력"=w475:errorcluster)  [unwired: 6 in, 2 out]
              n138 = call "Variables Data IO.vi"("Select"=Cmd_Var_Data_IO."Result3", "error in"=w475, "Func_ext"=w474) -> ("error out"=w472:errorcluster, "Data Out"=w466:string[][], "Func_ext Out"=w473:string)  [unwired: 6 in]
              n139 = call-poly "Table Initialize.vi"("Table Ref"=w470, "Value"=w466, "에러 입력"=w472) -> ("에러 출력"=w471:errorcluster)  [unwired: 6 in, 2 out]
              n140 = call "Enq Msg.vi"("에러 입력(에러 없음)"=w471, "메세지"="Value Change", "큐 입력"=w484) -> ("에러 출력"=w485:errorcluster)  [unwired: 7 in, 1 out]
            }
          }
        }
      }
    }
    frame "Length_14" {
      n141 = Index Array(array=w497) -> (element #1=w498:refnum<vi>, element #2=w499:refnum<vi>)  [unwired: 2 in]
      n142 = case shown="참" w492 {
        tunnel: [w501 w519] -> w494
        tunnel: w490 -> [w502 w522]
        tunnel: w498 -> [w505 w516]
        tunnel: w493 -> [w500 w512]
        tunnel: w496 -> [_ w518]
        tunnel: w495 -> [w506 w517]
        tunnel: w499 -> [w503 w515]
        tunnel: [w502 w514] -> w491
        frame False {
          n143 = call-poly "Table Initialize.vi"("행의 개수"=w500, "Table Ref"=w505, "에러 입력"=w506) -> ("에러 출력"=w504:errorcluster)  [unwired: 6 in, 2 out]
          n144 = call-poly "Table Initialize.vi"("행의 개수"=w500, "Table Ref"=w503, "에러 입력"=w504) -> ("에러 출력"=w501:errorcluster)  [unwired: 6 in, 2 out]
        }
        frame True {
          n145 = call "Variables Data IO.vi"("Select"=Cmd_Var_Data_IO."Result", "error in"=w517, "Func_ext"=w522) -> ("error out"=w521:errorcluster, "Data Out"=w510:string[][], "Func_ext Out"=w514:string)  [unwired: 6 in]
          n146 = Delete From Array(array=w510, length=14 ("길이")) -> (deleted portion=w508:string[][], array with subset deleted=w507:string[][])  [unwired: 2 in]
          n147 = call-poly "Table Initialize.vi"("행의 개수"=w512, "Table Ref"=w516, "Value"=w507, "에러 입력"=w521) -> ("에러 출력"=w511:errorcluster)  [unwired: 5 in, 2 out]
          n148 = call-poly "Table Initialize.vi"("행의 개수"=w512, "Table Ref"=w515, "Value"=w508, "에러 입력"=w511) -> ("에러 출력"=w513:errorcluster)  [unwired: 5 in, 2 out]
          n149 = call "Enq Msg.vi"("에러 입력(에러 없음)"=w513, "메세지"="Value Change", "큐 입력"=w518) -> ("에러 출력"=w519:errorcluster)  [unwired: 7 in, 1 out]
        }
      }
    }
    frame "Length_15" {
      n150 = Index Array(array=w539) -> (element #1=w533:refnum<vi>, element #2=w538:refnum<vi>)  [unwired: 2 in]
      n151 = Index Array(array=w540) -> (element=w536:refnum<vi>)  [unwired: 1 in]
      n152 = Index Array(array=w527, index (col)=5 ("비활성화된 인덱스 (열)")) -> (element=w529:string[])  [unwired: 1 in]
      n153 = property class="Tbl (엄격한)"(reference=w533, error in=w535) -> (reference out=w532:refnum<vi>, error out=w534:errorcluster, "Number of Rows"=w531:u32)
      n154 = Decimal String To Number(string=w529) -> (number=w526:i32[])  [unwired: 2 in, 1 out]
      n155 = Decrement(x=w531) -> (x-1=w530:u32)
      n156 = for {
        N: w530 -> [_]
        shift-right: [w553] -> w537
        shift-left: w534 -> [w554]
        tunnel: w532 -> [w552]
        tunnel: w526 -> [w550]
        tunnel: w536 -> [w548]
        tunnel: [w547] -> w525 mode=indexing
        tunnel: w524 -> [w546]
        i -> [w549]
        n157 = for {
          N: 8 -> [_]
          shift-right: [w570] -> w553
          shift-left: w554 -> [w579]
          tunnel: w552 -> [w578]
          tunnel: w549 -> [w566]
          tunnel: w550 -> [w575]
          tunnel: w549 -> [w562]
          tunnel: w548 -> [w568]
          tunnel: [w556] -> w547 mode=indexing
          tunnel: w546 -> [w555]
          i -> [w574]
          n158 = case shown="0, 1, 기본" w574 {
            tunnel: [2 0 1] -> w573
            frame 0, 1, Default {
            }
            frame 2, 3, 6 {
            }
            frame 4, 5, 7 {
            }
          }
          n159 = Bundle(w566, w574) -> (w569:cluster{i32, i32})  [unwired: 1 in]
          n160 = Index Array(array=w575, index=w573) -> (element=w572:i32)
          n161 = Greater?(x=w562, y=w572) -> (0:w560:bool)
          n162 = Equal To 0?(x=w562) -> (x = 0?=w559:bool)
          n163 = Or(x=w560, y=w559) -> (x .or. y?=w561:bool)
          n164 = Select(t="ⅹ", s=w560, f="") -> (s? t:f=w557:string)
          n165 = Select(t=u32 13816530, s=w561, f=u32 16448250) -> (s? t:f=w567:u32)
          n166 = property class="Tbl (엄격한)"(reference=w578, error in=w579, "Active Cell"=w569, "Cell BG Color"=w567) -> (error out=w571:errorcluster)  [unwired: 1 out]
          n167 = Select(t="-", s=w559, f=w557) -> (s? t:f=w556:string)
          n168 = property class="Tbl (엄격한)"(reference=w568, error in=w571, "Active Cell"=w569, "Cell BG Color"=w567, "Value"=string[][] [] ("값"), "Number of Rows"=w555) -> (error out=w570:errorcluster)  [unwired: 1 out]
        }
      }
      n169 = case shown="참" w543 {
        tunnel: [w585 w610] -> w544
        tunnel: w541 -> [w590 w600]
        tunnel: w524 -> [w584 w597]
        tunnel: w545 -> [_ w609]
        tunnel: w537 -> [w589 w596]
        tunnel: w533 -> [w587 w608]
        tunnel: [w590 w606] -> w542
        tunnel: w538 -> [w588 w598]
        tunnel: w525 -> [w583 _]
        frame False {
          n170 = call-poly "Table Initialize.vi"("Table Ref"=w588, "에러 입력"=w589) -> ("에러 출력"=w586:errorcluster)  [unwired: 7 in, 2 out]
          n171 = property class="Tbl (엄격한)"(reference=w587, error in=w586, "Number of Rows"=w584, "Value"=w583) -> (error out=w585:errorcluster)  [unwired: 1 out]
        }
        frame True {
          w592 = enum16{"행", "열", "행,열"}."행" ("조건")
          n172 = call "Variables Data IO.vi"("Select"=Cmd_Var_Data_IO."Result2", "error in"=w596, "Func_ext"=w600) -> ("error out"=w603:errorcluster, "Data Out"=w595:string[][], "Func_ext Out"=w599:string)  [unwired: 6 in]
          n173 = call-poly "Remove Empty Array.vi"("조건"=w592, "Data in"=w595) -> ("Data out"=w594:string[][])  [unwired: 8 in, 1 out]
          n174 = call-poly "Table Initialize.vi"("Table Ref"=w598, "Value"=w594, "에러 입력"=w603) -> ("에러 출력"=w602:errorcluster)  [unwired: 6 in, 2 out]
          n175 = call "Variables Data IO.vi"("Select"=Cmd_Var_Data_IO."Result", "error in"=w602, "Func_ext"=w599) -> ("error out"=w605:errorcluster, "Data Out"=w593:string[][], "Func_ext Out"=w606:string)  [unwired: 6 in]
          n176 = call-poly "Remove Empty Array.vi"("조건"=w592, "Data in"=w593) -> ("Data out"=w591:string[][])  [unwired: 8 in, 1 out]
          n177 = call-poly "Table Initialize.vi"("행의 개수"=w597, "Table Ref"=w608, "Value"=w591, "에러 입력"=w605) -> ("에러 출력"=w607:errorcluster)  [unwired: 5 in, 2 out]
          n178 = call "Enq Msg.vi"("에러 입력(에러 없음)"=w607, "메세지"="Value Change", "큐 입력"=w609) -> ("에러 출력"=w610:errorcluster)  [unwired: 7 in, 1 out]
        }
      }
    }
    frame "Length_2" {
      n179 = Index Array(array=w619) -> (element #1=w620:refnum<vi>, element #2=w621:refnum<vi>, element #3=w622:refnum<vi>)  [unwired: 3 in]
      n180 = case shown="참" w615 {
        tunnel: [w624 w649] -> w614
        tunnel: w612 -> [w623 w652]
        tunnel: w620 -> [w627 w645]
        tunnel: w616 -> [w629 w648]
        tunnel: w618 -> [_ w647]
        tunnel: w617 -> [w628 w646]
        tunnel: w621 -> [w625 w641]
        tunnel: w622 -> [_ w634]
        tunnel: [w623 w633] -> w613
        frame False {
          n181 = call-poly "Table Initialize.vi"("행의 개수"=w629, "Table Ref"=w627, "에러 입력"=w628) -> ("에러 출력"=w626:errorcluster)  [unwired: 6 in, 2 out]
          n182 = call-poly "Table Initialize.vi"("Table Ref"=w625, "에러 입력"=w626) -> ("에러 출력"=w624:errorcluster)  [unwired: 7 in, 2 out]
        }
        frame True {
          n183 = call "Variables Data IO.vi"("Select"=Cmd_Var_Data_IO."Result", "error in"=w646, "Func_ext"=w652) -> ("error out"=w651:errorcluster, "Data Out"=w632:string[][], "Func_ext Out"=w640:string)  [unwired: 6 in]
          n184 = call-poly "Table Initialize.vi"("행의 개수"=w648, "Table Ref"=w645, "Value"=w632, "에러 입력"=w651) -> ("에러 출력"=w642:errorcluster)  [unwired: 5 in, 2 out]
          n185 = call "Variables Data IO.vi"("Select"=Cmd_Var_Data_IO."Result2", "error in"=w642, "Func_ext"=w640) -> ("error out"=w644:errorcluster, "Data Out"=w631:string[][], "Func_ext Out"=w635:string)  [unwired: 6 in]
          n186 = call-poly "Table Initialize.vi"("Table Ref"=w641, "Value"=w631, "에러 입력"=w644) -> ("에러 출력"=w638:errorcluster)  [unwired: 6 in, 2 out]
          n187 = call "Variables Data IO.vi"("Select"=Cmd_Var_Data_IO."Result3", "error in"=w638, "Func_ext"=w635) -> ("error out"=w639:errorcluster, "Data Out"=w630:string[][], "Func_ext Out"=w633:string)  [unwired: 6 in]
          n188 = call-poly "Table Initialize.vi"("Table Ref"=w634, "Value"=w630, "에러 입력"=w639) -> ("에러 출력"=w637:errorcluster)  [unwired: 6 in, 2 out]
          n189 = call "Enq Msg.vi"("에러 입력(에러 없음)"=w637, "메세지"="Value Change", "큐 입력"=w647) -> ("에러 출력"=w649:errorcluster)  [unwired: 7 in, 1 out]
        }
      }
    }
    frame "Length_3" {
      n190 = Index Array(array=w657) -> (element=w656:refnum<vi>)  [unwired: 1 in]
      n191 = Index Array(array=w665) -> (element #1=w666:refnum<vi>, element #2=w655:refnum<vi>)  [unwired: 2 in]
      n192 = case shown="거짓" w660 {
        tunnel: [w669 w700] -> w662
        tunnel: w658 -> [w672 w703]
        tunnel: w666 -> [w675 w696]
        tunnel: w661 -> [w668 w699]
        tunnel: w664 -> [_ w698]
        tunnel: w663 -> [w676 w697]
        tunnel: w655 -> [w673 w692]
        tunnel: [w672 w686] -> w659
        tunnel: w656 -> [w671 w685]
        tunnel: w654 -> [w667 _]
        frame False {
          n193 = call-poly "Table Initialize.vi"("행의 개수"=w668, "Table Ref"=w675, "에러 입력"=w676) -> ("에러 출력"=w674:errorcluster)  [unwired: 6 in, 2 out]
          n194 = case shown="\"10517-0\"" w667 {
            tunnel: w674 -> [w677 w680]
            tunnel: w673 -> [_ w679]
            tunnel: [w677 w678] -> w670
            frame "10517-0" {
            }
            frame Default {
              n195 = call-poly "Table Initialize.vi"("Table Ref"=w679, "에러 입력"=w680) -> ("에러 출력"=w678:errorcluster)  [unwired: 7 in, 2 out]
            }
          }
          n196 = call-poly "Table Initialize.vi"("행의 개수"=w668, "Table Ref"=w671, "에러 입력"=w670) -> ("에러 출력"=w669:errorcluster)  [unwired: 6 in, 2 out]
        }
        frame True {
          n197 = call "Variables Data IO.vi"("Select"=Cmd_Var_Data_IO."Result", "error in"=w697, "Func_ext"=w703) -> ("error out"=w702:errorcluster, "Data Out"=w683:string[][], "Func_ext Out"=w691:string)  [unwired: 6 in]
          n198 = call-poly "Table Initialize.vi"("행의 개수"=w699, "Table Ref"=w696, "Value"=w683, "에러 입력"=w702) -> ("에러 출력"=w693:errorcluster)  [unwired: 5 in, 2 out]
          n199 = call "Variables Data IO.vi"("Select"=Cmd_Var_Data_IO."Result2", "error in"=w693, "Func_ext"=w691) -> ("error out"=w695:errorcluster, "Data Out"=w682:string[][], "Func_ext Out"=w687:string)  [unwired: 6 in]
          n200 = call-poly "Table Initialize.vi"("Table Ref"=w692, "Value"=w682, "에러 입력"=w695) -> ("에러 출력"=w689:errorcluster)  [unwired: 6 in, 2 out]
          n201 = call "Variables Data IO.vi"("Select"=Cmd_Var_Data_IO."Result_ADJ", "error in"=w689, "Func_ext"=w687) -> ("error out"=w690:errorcluster, "Data Out"=w681:string[][], "Func_ext Out"=w686:string)  [unwired: 6 in]
          n202 = call-poly "Table Initialize.vi"("Table Ref"=w685, "Value"=w681, "에러 입력"=w690) -> ("에러 출력"=w688:errorcluster)  [unwired: 6 in, 2 out]
          n203 = call "Enq Msg.vi"("에러 입력(에러 없음)"=w688, "메세지"="Value Change", "큐 입력"=w698) -> ("에러 출력"=w700:errorcluster)  [unwired: 7 in, 1 out]
        }
      }
    }
    frame "Length_4" {
      n204 = Index Array(array=w707) -> (element=w706:refnum<vi>)  [unwired: 1 in]
      n205 = case shown="참" w713 {
        tunnel: [w716 w735] -> w710
        tunnel: w705 -> [w715 w728]
        tunnel: w706 -> [w717 w732]
        tunnel: w712 -> [w719 w734]
        tunnel: w711 -> [_ w733]
        tunnel: w714 -> [w718 w729]
        tunnel: w708 -> [_ w722]
        tunnel: [w715 w721] -> w709
        frame False {
          n206 = call-poly "Table Initialize.vi"("행의 개수"=w719, "Table Ref"=w717, "에러 입력"=w718) -> ("에러 출력"=w716:errorcluster)  [unwired: 6 in, 2 out]
        }
        frame True {
          n207 = call "Variables Data IO.vi"("Select"=Cmd_Var_Data_IO."Result2", "error in"=w729, "Func_ext"=w728) -> ("error out"=w726:errorcluster, "Data Out"=w724:string[][], "Func_ext Out"=w727:string)  [unwired: 6 in]
          n208 = Index Array(array=w724) -> (element=w723:string[])  [unwired: 2 in]
          n209 = for {
            shift-right: [w741] -> w725
            shift-left: w726 -> [w742]
            tunnel: w723 -> [w740] mode=indexing
            tunnel: w722 -> [w739] mode=indexing
            n210 = property class="CmbBox"(reference=w739, error in=w742, "Value"=w740) -> (error out=w741:errorcluster)  [unwired: 1 out]
          }
          n211 = call "Variables Data IO.vi"("Select"=Cmd_Var_Data_IO."Result", "error in"=w725, "Func_ext"=w727) -> ("error out"=w737:errorcluster, "Data Out"=w720:string[][], "Func_ext Out"=w721:string)  [unwired: 6 in]
          n212 = call-poly "Table Initialize.vi"("행의 개수"=w734, "Table Ref"=w732, "Value"=w720, "에러 입력"=w737) -> ("에러 출력"=w731:errorcluster)  [unwired: 5 in, 2 out]
          n213 = call "Enq Msg.vi"("에러 입력(에러 없음)"=w731, "메세지"="Value Change", "큐 입력"=w733) -> ("에러 출력"=w735:errorcluster)  [unwired: 7 in, 1 out]
        }
      }
    }
    frame "Length_6_1" {
      n214 = Index Array(array=w753) -> (element #1=w754:refnum<vi>, element #2=w755:refnum<vi>)  [unwired: 2 in]
      n215 = Index Array(array=w745) -> (element=w744:refnum<vi>)  [unwired: 1 in]
      n216 = case shown="기본" w743 {
        tunnel: w755 -> [w765 w808 w851]
        tunnel: w754 -> [w764 w807 w850]
        tunnel: w752 -> [w763 w806 w849]
        tunnel: w751 -> [w762 w805 w848]
        tunnel: [w761 w804 w847] -> w750
        tunnel: w749 -> [w760 w803 w846]
        tunnel: w748 -> [w759 w802 w845]
        tunnel: [w758 w801 w844] -> w747
        tunnel: w746 -> [w757 w800 w843]
        tunnel: w744 -> [w756 w799 w842]
        frame Default {
          n217 = case shown="참" w759 {
            tunnel: [w768 w794] -> w761
            tunnel: w757 -> [w770 w797]
            tunnel: w764 -> [w773 w791]
            tunnel: w760 -> [w766 w778]
            tunnel: w763 -> [_ w793]
            tunnel: w762 -> [w774 w792]
            tunnel: w765 -> [w771 w787]
            tunnel: [w770 w782] -> w758
            tunnel: w756 -> [w767 w780]
            frame False {
              n218 = call-poly "Table Initialize.vi"("행의 개수"=w766, "Table Ref"=w773, "에러 입력"=w774) -> ("에러 출력"=w772:errorcluster)  [unwired: 6 in, 2 out]
              n219 = call-poly "Table Initialize.vi"("행의 개수"=w766, "Table Ref"=w771, "에러 입력"=w772) -> ("에러 출력"=w769:errorcluster)  [unwired: 6 in, 2 out]
              n220 = call-poly "Table Initialize.vi"("행의 개수"=w766, "Table Ref"=w767, "에러 입력"=w769) -> ("에러 출력"=w768:errorcluster)  [unwired: 6 in, 2 out]
            }
            frame True {
              n221 = call "Variables Data IO.vi"("Select"=Cmd_Var_Data_IO."Result", "error in"=w792, "Func_ext"=w797) -> ("error out"=w796:errorcluster, "Data Out"=w777:string[][], "Func_ext Out"=w786:string)  [unwired: 6 in]
              n222 = call-poly "Table Initialize.vi"("행의 개수"=w778, "Table Ref"=w791, "Value"=w777, "에러 입력"=w796) -> ("에러 출력"=w788:errorcluster)  [unwired: 5 in, 2 out]
              n223 = call "Variables Data IO.vi"("Select"=Cmd_Var_Data_IO."Result2", "error in"=w788, "Func_ext"=w786) -> ("error out"=w790:errorcluster, "Data Out"=w776:string[][], "Func_ext Out"=w783:string)  [unwired: 6 in]
              n224 = call-poly "Table Initialize.vi"("행의 개수"=w778, "Table Ref"=w787, "Value"=w776, "에러 입력"=w790) -> ("에러 출력"=w785:errorcluster)  [unwired: 5 in, 2 out]
              n225 = call "Variables Data IO.vi"("Select"=Cmd_Var_Data_IO."Result3", "error in"=w785, "Func_ext"=w783) -> ("error out"=w779:errorcluster, "Data Out"=w775:string[][], "Func_ext Out"=w782:string)  [unwired: 6 in]
              n226 = call-poly "Table Initialize.vi"("행의 개수"=w778, "Table Ref"=w780, "Value"=w775, "에러 입력"=w779) -> ("에러 출력"=w784:errorcluster)  [unwired: 5 in, 2 out]
              n227 = call "Enq Msg.vi"("에러 입력(에러 없음)"=w784, "메세지"="Value Change", "큐 입력"=w793) -> ("에러 출력"=w794:errorcluster)  [unwired: 7 in, 1 out]
            }
          }
        }
        frame "10405-0" {
          n228 = case shown="참" w802 {
            tunnel: [w811 w837] -> w804
            tunnel: w800 -> [w813 w840]
            tunnel: w807 -> [w816 w834]
            tunnel: w803 -> [w809 w821]
            tunnel: w806 -> [_ w836]
            tunnel: w805 -> [w817 w835]
            tunnel: w808 -> [w814 w830]
            tunnel: [w813 w825] -> w801
            tunnel: w799 -> [w810 w823]
            frame False {
              n229 = call-poly "Table Initialize.vi"("행의 개수"=w809, "Table Ref"=w816, "에러 입력"=w817) -> ("에러 출력"=w815:errorcluster)  [unwired: 6 in, 2 out]
              n230 = call-poly "Table Initialize.vi"("행의 개수"=w809, "Table Ref"=w814, "에러 입력"=w815) -> ("에러 출력"=w812:errorcluster)  [unwired: 6 in, 2 out]
              n231 = call-poly "Table Initialize.vi"("Table Ref"=w810, "에러 입력"=w812) -> ("에러 출력"=w811:errorcluster)  [unwired: 7 in, 2 out]
            }
            frame True {
              n232 = call "Variables Data IO.vi"("Select"=Cmd_Var_Data_IO."Result", "error in"=w835, "Func_ext"=w840) -> ("error out"=w839:errorcluster, "Data Out"=w818:string[][], "Func_ext Out"=w829:string)  [unwired: 6 in]
              n233 = call-poly "Table Initialize.vi"("행의 개수"=w821, "Table Ref"=w834, "Value"=w818, "에러 입력"=w839) -> ("에러 출력"=w831:errorcluster)  [unwired: 5 in, 2 out]
              n234 = call "Variables Data IO.vi"("Select"=Cmd_Var_Data_IO."Result2", "error in"=w831, "Func_ext"=w829) -> ("error out"=w833:errorcluster, "Data Out"=w819:string[][], "Func_ext Out"=w826:string)  [unwired: 6 in]
              n235 = call-poly "Table Initialize.vi"("행의 개수"=w821, "Table Ref"=w830, "Value"=w819, "에러 입력"=w833) -> ("에러 출력"=w828:errorcluster)  [unwired: 5 in, 2 out]
              n236 = call "Variables Data IO.vi"("Select"=Cmd_Var_Data_IO."Result3", "error in"=w828, "Func_ext"=w826) -> ("error out"=w822:errorcluster, "Data Out"=w820:string[][], "Func_ext Out"=w825:string)  [unwired: 6 in]
              n237 = call-poly "Table Initialize.vi"("Table Ref"=w823, "Value"=w820, "에러 입력"=w822) -> ("에러 출력"=w827:errorcluster)  [unwired: 6 in, 2 out]
              n238 = call "Enq Msg.vi"("에러 입력(에러 없음)"=w827, "메세지"="Value Change", "큐 입력"=w836) -> ("에러 출력"=w837:errorcluster)  [unwired: 7 in, 1 out]
            }
          }
        }
        frame "10404-0" {
          n239 = case shown="참" w845 {
            tunnel: [w855 w873] -> w847
            tunnel: w843 -> [w854 w876]
            tunnel: w850 -> [w858 w870]
            tunnel: w846 -> [w853 w869]
            tunnel: w849 -> [_ w872]
            tunnel: w848 -> [w859 w871]
            tunnel: w851 -> [w856 _]
            tunnel: [w854 w862] -> w844
            tunnel: w842 -> [_ w865]
            frame False {
              n240 = call-poly "Table Initialize.vi"("행의 개수"=w853, "Table Ref"=w858, "에러 입력"=w859) -> ("에러 출력"=w857:errorcluster)  [unwired: 6 in, 2 out]
              n241 = call-poly "Table Initialize.vi"("행의 개수"=w853, "Table Ref"=w856, "비활성화?"=TRUE, "에러 입력"=w857) -> ("에러 출력"=w855:errorcluster)  [unwired: 5 in, 2 out]
            }
            frame True {
              n242 = call "Variables Data IO.vi"("Select"=Cmd_Var_Data_IO."Result", "error in"=w871, "Func_ext"=w876) -> ("error out"=w875:errorcluster, "Data Out"=w861:string[][], "Func_ext Out"=w863:string)  [unwired: 6 in]
              n243 = call-poly "Table Initialize.vi"("행의 개수"=w869, "Table Ref"=w870, "Value"=w861, "에러 입력"=w875) -> ("에러 출력"=w868:errorcluster)  [unwired: 5 in, 2 out]
              n244 = call "Variables Data IO.vi"("Select"=Cmd_Var_Data_IO."Result3", "error in"=w868, "Func_ext"=w863) -> ("error out"=w866:errorcluster, "Data Out"=w860:string[][], "Func_ext Out"=w862:string)  [unwired: 6 in]
              n245 = call-poly "Table Initialize.vi"("Table Ref"=w865, "Value"=w860, "에러 입력"=w866) -> ("에러 출력"=w867:errorcluster)  [unwired: 6 in, 2 out]
              n246 = call "Enq Msg.vi"("에러 입력(에러 없음)"=w867, "메세지"="Value Change", "큐 입력"=w872) -> ("에러 출력"=w873:errorcluster)  [unwired: 7 in, 1 out]
            }
          }
        }
      }
    }
    frame "Length_9" {
      n247 = Index Array(array=w885) -> (element #1=w886:refnum<vi>, element #2=w887:refnum<vi>)  [unwired: 2 in]
      n248 = case shown="참" w880 {
        tunnel: [w890 w902] -> w882
        tunnel: w878 -> [w889 w905]
        tunnel: w886 -> [w893 w898]
        tunnel: w881 -> [w888 w901]
        tunnel: w884 -> [_ w900]
        tunnel: w883 -> [w894 w899]
        tunnel: w887 -> [w891 _]
        tunnel: [w889 w896] -> w879
        frame False {
          n249 = call-poly "Table Initialize.vi"("행의 개수"=w888, "Table Ref"=w893, "에러 입력"=w894) -> ("에러 출력"=w892:errorcluster)  [unwired: 6 in, 2 out]
          n250 = call-poly "Table Initialize.vi"("행의 개수"=w888, "Table Ref"=w891, "에러 입력"=w892) -> ("에러 출력"=w890:errorcluster)  [unwired: 6 in, 2 out]
        }
        frame True {
          n251 = call "Variables Data IO.vi"("Select"=Cmd_Var_Data_IO."Result", "error in"=w899, "Func_ext"=w905) -> ("error out"=w904:errorcluster, "Data Out"=w895:string[][], "Func_ext Out"=w896:string)  [unwired: 6 in]
          n252 = call-poly "Table Initialize.vi"("행의 개수"=w901, "Table Ref"=w898, "Value"=w895, "에러 입력"=w904) -> ("에러 출력"=w897:errorcluster)  [unwired: 5 in, 2 out]
          n253 = call "Enq Msg.vi"("에러 입력(에러 없음)"=w897, "메세지"="Value Change", "큐 입력"=w900) -> ("에러 출력"=w902:errorcluster)  [unwired: 7 in, 1 out]
        }
      }
    }
    frame "Mass_1_1", "Mass_1_2", "Mass_1_3" {
      n254 = Index Array(array=w912) -> (element=w911:refnum<vi>)  [unwired: 1 in]
      n255 = Index Array(array=w908) -> (element=w907:refnum<vi>)  [unwired: 1 in]
      n256 = Index Array(array=w918) -> (element=w919:refnum<vi>)  [unwired: 1 in]
      n257 = case shown="참" w913 {
        tunnel: [w922 w949] -> w915
        tunnel: w909 -> [w924 w952]
        tunnel: w919 -> [w927 w946]
        tunnel: w914 -> [w920 w934]
        tunnel: w917 -> [_ w948]
        tunnel: w916 -> [w928 w947]
        tunnel: w911 -> [w925 w942]
        tunnel: [w924 w935] -> w910
        tunnel: w907 -> [w921 w932]
        frame False {
          n258 = call-poly "Table Initialize.vi"("행의 개수"=w920, "Table Ref"=w927, "에러 입력"=w928) -> ("에러 출력"=w926:errorcluster)  [unwired: 6 in, 2 out]
          n259 = call-poly "Table Initialize.vi"("Table Ref"=w925, "에러 입력"=w926) -> ("에러 출력"=w923:errorcluster)  [unwired: 7 in, 2 out]
          n260 = call-poly "Table Initialize.vi"("행의 개수"=w920, "Table Ref"=w921, "에러 입력"=w923) -> ("에러 출력"=w922:errorcluster)  [unwired: 6 in, 2 out]
        }
        frame True {
          n261 = call "Variables Data IO.vi"("Select"=Cmd_Var_Data_IO."Result", "error in"=w947, "Func_ext"=w952) -> ("error out"=w951:errorcluster, "Data Out"=w929:string[][], "Func_ext Out"=w941:string)  [unwired: 6 in]
          n262 = call-poly "Table Initialize.vi"("행의 개수"=w934, "Table Ref"=w946, "Value"=w929, "에러 입력"=w951) -> ("에러 출력"=w943:errorcluster)  [unwired: 5 in, 2 out]
          n263 = call "Variables Data IO.vi"("Select"=Cmd_Var_Data_IO."Result2", "error in"=w943, "Func_ext"=w941) -> ("error out"=w945:errorcluster, "Data Out"=w930:string[][], "Func_ext Out"=w936:string)  [unwired: 6 in]
          n264 = call-poly "Table Initialize.vi"("행의 개수"=u32 3, "Table Ref"=w942, "Value"=w930, "에러 입력"=w945) -> ("에러 출력"=w938:errorcluster)  [unwired: 5 in, 2 out]
          n265 = call "Variables Data IO.vi"("Select"=Cmd_Var_Data_IO."Result_ADJ", "error in"=w938, "Func_ext"=w936) -> ("error out"=w939:errorcluster, "Data Out"=w931:string[][], "Func_ext Out"=w935:string)  [unwired: 6 in]
          n266 = call-poly "Table Initialize.vi"("행의 개수"=w934, "Table Ref"=w932, "Value"=w931, "에러 입력"=w939) -> ("에러 출력"=w937:errorcluster)  [unwired: 5 in, 2 out]
          n267 = call "Enq Msg.vi"("에러 입력(에러 없음)"=w937, "메세지"="Value Change", "큐 입력"=w948) -> ("에러 출력"=w949:errorcluster)  [unwired: 7 in, 1 out]
        }
      }
    }
    frame "Pressure_1", "Pressure_3" {
      n268 = case shown="\"Check\"" w958 {
        tunnel: [_ TRUE] -> w957
        frame Default {
        }
        frame "Check" {
        }
      }
      n269 = Index Array(array=w955) -> (element=w954:refnum<vi>)  [unwired: 1 in]
      n270 = Index Array(array=w967) -> (element #1=w966:refnum<vi>, element #2=w965:refnum<vi>)  [unwired: 2 in]
      n271 = case shown="참" w964 {
        tunnel: w966 -> [w978 w993]
        tunnel: w957 -> [w971 w984]
        tunnel: [w974 w995] -> w959
        tunnel: w962 -> [w972 w985]
        tunnel: w965 -> [w977 w992]
        tunnel: w961 -> [w970 w982]
        tunnel: w963 -> [w980 w999]
        tunnel: w956 -> [w976 w998]
        tunnel: w968 -> [_ w994]
        tunnel: [w976 w989] -> w960
        tunnel: w954 -> [w973 w986]
        frame False {
          n272 = call-poly "Table Initialize.vi"("행의 개수"=w972, "Table Ref"=w978, "Value"=w970, "비활성화?"=w971, "에러 입력"=w980) -> ("에러 출력"=w979:errorcluster)  [unwired: 4 in, 2 out]
          n273 = call-poly "Table Initialize.vi"("Table Ref"=w977, "Value"=w970, "에러 입력"=w979) -> ("에러 출력"=w975:errorcluster)  [unwired: 6 in, 2 out]
          n274 = call-poly "Table Initialize.vi"("행의 개수"=w972, "Table Ref"=w973, "Value"=w970, "비활성화?"=w971, "에러 입력"=w975) -> ("에러 출력"=w974:errorcluster)  [unwired: 4 in, 2 out]
        }
        frame True {
          n275 = call "Variables Data IO.vi"("Select"=Cmd_Var_Data_IO."Result", "error in"=w999, "Func_ext"=w998) -> ("error out"=w997:errorcluster, "Data Out"=w983:string[][], "Func_ext Out"=w990:string)  [unwired: 6 in]
          n276 = call-poly "Table Initialize.vi"("행의 개수"=w985, "Table Ref"=w993, "Value"=w983, "비활성화?"=w984, "에러 입력"=w997) -> ("에러 출력"=w1002:errorcluster)  [unwired: 4 in, 2 out]
          n277 = call-poly "Table Initialize.vi"("Table Ref"=w992, "Value"=w982, "에러 입력"=w1002) -> ("에러 출력"=w1001:errorcluster)  [unwired: 6 in, 2 out]
          n278 = call "Variables Data IO.vi"("Select"=Cmd_Var_Data_IO."Result_ADJ", "error in"=w1001, "Func_ext"=w990) -> ("error out"=w988:errorcluster, "Data Out"=w981:string[][], "Func_ext Out"=w989:string)  [unwired: 6 in]
          n279 = call-poly "Table Initialize.vi"("행의 개수"=w985, "Table Ref"=w986, "Value"=w981, "비활성화?"=w984, "에러 입력"=w988) -> ("에러 출력"=w987:errorcluster)  [unwired: 4 in, 2 out]
          n280 = call "Enq Msg.vi"("에러 입력(에러 없음)"=w987, "메세지"="Value Change", "큐 입력"=w994) -> ("에러 출력"=w995:errorcluster)  [unwired: 7 in, 1 out]
        }
      }
    }
    frame "Pressure_2" {
      n281 = Index Array(array=w1004) -> (element=w1003:refnum<vi>)  [unwired: 1 in]
      n282 = Index Array(array=w1014) -> (element #1=w1013:refnum<vi>, element #2=w1012:refnum<vi>)  [unwired: 2 in]
      n283 = case shown="참" w1011 {
        tunnel: w1013 -> [w1023 w1038]
        tunnel: [w1020 w1040] -> w1006
        tunnel: w1009 -> [w1018 w1032]
        tunnel: w1012 -> [w1022 w1037]
        tunnel: w1008 -> [w1016 w1028]
        tunnel: w1010 -> [w1025 w1044]
        tunnel: w1005 -> [w1021 w1043]
        tunnel: w1015 -> [_ w1039]
        tunnel: [w1021 w1033] -> w1007
        tunnel: w1003 -> [w1019 w1031]
        frame False {
          n284 = call-poly "Table Initialize.vi"("행의 개수"=w1018, "Table Ref"=w1023, "Value"=w1016, "에러 입력"=w1025) -> ("에러 출력"=w1024:errorcluster)  [unwired: 5 in, 2 out]
          n285 = call-poly "Table Initialize.vi"("Table Ref"=w1022, "Value"=w1016, "에러 입력"=w1024) -> ("에러 출력"=w1017:errorcluster)  [unwired: 6 in, 2 out]
          n286 = call-poly "Table Initialize.vi"("행의 개수"=w1018, "Table Ref"=w1019, "Value"=w1016, "에러 입력"=w1017) -> ("에러 출력"=w1020:errorcluster)  [unwired: 5 in, 2 out]
        }
        frame True {
          n287 = call "Variables Data IO.vi"("Select"=Cmd_Var_Data_IO."Result", "error in"=w1044, "Func_ext"=w1043) -> ("error out"=w1042:errorcluster, "Data Out"=w1027:string[][], "Func_ext Out"=w1034:string)  [unwired: 6 in]
          n288 = call-poly "Table Initialize.vi"("행의 개수"=w1032, "Table Ref"=w1038, "Value"=w1027, "에러 입력"=w1042) -> ("에러 출력"=w1046:errorcluster)  [unwired: 5 in, 2 out]
          n289 = call-poly "Table Initialize.vi"("Table Ref"=w1037, "Value"=w1028, "에러 입력"=w1046) -> ("에러 출력"=w1030:errorcluster)  [unwired: 6 in, 2 out]
          n290 = call "Variables Data IO.vi"("Select"=Cmd_Var_Data_IO."Result_ADJ", "error in"=w1030, "Func_ext"=w1034) -> ("error out"=w1036:errorcluster, "Data Out"=w1026:string[][], "Func_ext Out"=w1033:string)  [unwired: 6 in]
          n291 = call-poly "Table Initialize.vi"("행의 개수"=w1032, "Table Ref"=w1031, "Value"=w1026, "에러 입력"=w1036) -> ("에러 출력"=w1029:errorcluster)  [unwired: 5 in, 2 out]
          n292 = call "Enq Msg.vi"("에러 입력(에러 없음)"=w1029, "메세지"="Value Change", "큐 입력"=w1039) -> ("에러 출력"=w1040:errorcluster)  [unwired: 7 in, 1 out]
        }
      }
    }
    frame "Torque_1", "Torque_2" {
      n293 = Index Array(array=w1061) -> (element=w1060:refnum<vi>)  [unwired: 1 in]
      n294 = property on="측정방향" class="Enum"(reference=w1060, error in=w1059) -> (error out=w1058:errorcluster, "Value"=w1057:variant)  [unwired: 1 out]
      n295 = Variant To Data(error in=w1058, type=enum16{"양방향", "시계방향", "반시계방향"}."양방향" ("측정방향 2"), Variant=w1057) -> (data=w1049:enum16{"양방향", "시계방향", "반시계방향"}, error out=w1055:errorcluster)
      n296 = case shown="\"반시계방향\"" w1049 {
        tunnel: [w1065 w1068 w1071] -> w1048
        frame "양방향", Default {
          w1064 = FALSE
          n297 = Build Array(w1064, w1064) -> (w1065:bool[])
        }
        frame "시계방향" {
          n298 = Build Array(FALSE, TRUE ("원소")) -> (w1068:bool[])
        }
        frame "반시계방향" {
          n299 = Build Array(TRUE, FALSE ("원소")) -> (w1071:bool[])
        }
      }
      n300 = case shown="거짓" w1062 {
        tunnel: w1055 -> [w1080 w1102]
        tunnel: [w1075 w1106] -> w1052
        tunnel: w1051 -> [w1079 w1103]
        tunnel: w1054 -> [w1072 w1096]
        tunnel: w1063 -> [_ w1105]
        tunnel: [w1079 w1093] -> w1053
        tunnel: w1050 -> [w1078 w1101]
        tunnel: w1048 -> [w1077 w1092]
        tunnel: w1047 -> [w1074 w1095]
        frame False {
          n301 = for {
            tunnel: w1072 -> [w1089]
            shift-right: [w1088] -> w1076
            shift-left: w1080 -> [w1090]
            tunnel: w1077 -> [w1086] mode=indexing
            tunnel: w1078 -> [w1087] mode=indexing
            tunnel: [w1086] -> w1073 mode=indexing
            n302 = call-poly "Table Initialize.vi"("행의 개수"=w1089, "Table Ref"=w1087, "비활성화?"=w1086, "에러 입력"=w1090) -> ("에러 출력"=w1088:errorcluster)  [unwired: 5 in, 2 out]
          }
          n303 = for {
            tunnel: w1072 -> [w1084]
            shift-right: [w1083] -> w1075
            shift-left: w1076 -> [w1085]
            tunnel: w1073 -> [w1082] mode=indexing
            tunnel: w1074 -> [w1081] mode=indexing
            n304 = call-poly "Table Initialize.vi"("행의 개수"=w1084, "Table Ref"=w1081, "비활성화?"=w1082, "에러 입력"=w1085) -> ("에러 출력"=w1083:errorcluster)  [unwired: 5 in, 2 out]
          }
        }
        frame True {
          w1099 = T3[] [enum."Result_ADJ", enum."Result_ADJ2"] items=["Condition", "Condition Default", "Condition_Temp", "Resolution", "Resolution Default", "Resolution Old", "Spec", "Spec Default", "Spec Old", "Spec Temp", "Result", "Result2", "Result3", "Result_Temp", "Result_ADJ", "Result_ADJ2", "STD1", "STD2", "STD3", "STD4", "STD5", "STD Temp", "CMC", "CMC Default"]
          w1100 = T3[] [enum."Result", enum."Result2"] items=["Condition", "Condition Default", "Condition_Temp", "Resolution", "Resolution Default", "Resolution Old", "Spec", "Spec Default", "Spec Old", "Spec Temp", "Result", "Result2", "Result3", "Result_Temp", "Result_ADJ", "Result_ADJ2", "STD1", "STD2", "STD3", "STD4", "STD5", "STD Temp", "CMC", "CMC Default"]
          n305 = for {
            tunnel: w1101 -> [w1124] mode=indexing
            tunnel: w1096 -> [w1126]
            shift-right: [w1125] -> w1098
            shift-left: w1102 -> [w1120]
            tunnel: w1092 -> [w1118] mode=indexing
            tunnel: w1100 -> [w1123] mode=indexing
            tunnel: w1103 -> [w1122]
            tunnel: [w1121] -> w1094
            tunnel: [w1118] -> w1091 mode=indexing
            n306 = call "Variables Data IO.vi"("Select"=w1123, "error in"=w1120, "Func_ext"=w1122) -> ("error out"=w1119:errorcluster, "Data Out"=w1117:string[][], "Func_ext Out"=w1121:string)  [unwired: 6 in]
            n307 = call-poly "Table Initialize.vi"("행의 개수"=w1126, "Table Ref"=w1124, "Value"=w1117, "비활성화?"=w1118, "에러 입력"=w1119) -> ("에러 출력"=w1125:errorcluster)  [unwired: 4 in, 2 out]
          }
          n308 = for {
            tunnel: w1095 -> [w1113] mode=indexing
            tunnel: w1096 -> [w1116]
            shift-right: [w1115] -> w1097
            shift-left: w1098 -> [w1109]
            tunnel: w1091 -> [w1114] mode=indexing
            tunnel: w1099 -> [w1112] mode=indexing
            tunnel: w1094 -> [w1111]
            tunnel: [w1110] -> w1093
            n309 = call "Variables Data IO.vi"("Select"=w1112, "error in"=w1109, "Func_ext"=w1111) -> ("error out"=w1108:errorcluster, "Data Out"=w1107:string[][], "Func_ext Out"=w1110:string)  [unwired: 6 in]
            n310 = call-poly "Table Initialize.vi"("행의 개수"=w1116, "Table Ref"=w1113, "Value"=w1107, "비활성화?"=w1114, "에러 입력"=w1108) -> ("에러 출력"=w1115:errorcluster)  [unwired: 4 in, 2 out]
          }
          n311 = call "Enq Msg.vi"("에러 입력(에러 없음)"=w1097, "메세지"="Value Change", "큐 입력"=w1105) -> ("에러 출력"=w1106:errorcluster)  [unwired: 7 in, 1 out]
        }
      }
    }
    frame Default {
      n312 = Index Array(array=w1132) -> (element=w1131:refnum<vi>)  [unwired: 1 in]
      n313 = Index Array(array=w1128) -> (element=w1127:refnum<vi>)  [unwired: 1 in]
      n314 = case shown="참" w1134 {
        tunnel: w1133 -> [w1144 w1162]
        tunnel: [w1138 w1158] -> w1135
        tunnel: w1129 -> [w1142 w1160]
        tunnel: w1131 -> [w1143 w1156]
        tunnel: w1136 -> [w1139 w1153]
        tunnel: w1137 -> [_ w1157]
        tunnel: [w1142 w1150] -> w1130
        tunnel: w1127 -> [w1140 w1152]
        frame False {
          n315 = call-poly "Table Initialize.vi"("행의 개수"=w1139, "Table Ref"=w1143, "에러 입력"=w1144) -> ("에러 출력"=w1141:errorcluster)  [unwired: 6 in, 2 out]
          n316 = call-poly "Table Initialize.vi"("행의 개수"=w1139, "Table Ref"=w1140, "에러 입력"=w1141) -> ("에러 출력"=w1138:errorcluster)  [unwired: 6 in, 2 out]
        }
        frame True {
          n317 = call "Variables Data IO.vi"("Select"=Cmd_Var_Data_IO."Result", "error in"=w1162, "Func_ext"=w1160) -> ("error out"=w1146:errorcluster, "Data Out"=w1145:string[][], "Func_ext Out"=w1151:string)  [unwired: 6 in]
          n318 = call-poly "Table Initialize.vi"("행의 개수"=w1153, "Table Ref"=w1156, "Value"=w1145, "에러 입력"=w1146) -> ("에러 출력"=w1155:errorcluster)  [unwired: 5 in, 2 out]
          n319 = call "Variables Data IO.vi"("Select"=Cmd_Var_Data_IO."Result_ADJ", "error in"=w1155, "Func_ext"=w1151) -> ("error out"=w1149:errorcluster, "Data Out"=w1147:string[][], "Func_ext Out"=w1150:string)  [unwired: 6 in]
          n320 = call-poly "Table Initialize.vi"("행의 개수"=w1153, "Table Ref"=w1152, "Value"=w1147, "에러 입력"=w1149) -> ("에러 출력"=w1154:errorcluster)  [unwired: 5 in, 2 out]
          n321 = call "Enq Msg.vi"("에러 입력(에러 없음)"=w1154, "메세지"="Value Change", "큐 입력"=w1157) -> ("에러 출력"=w1158:errorcluster)  [unwired: 7 in, 1 out]
        }
      }
    }
    frame "Flatness_1" {
      n322 = Index Array(array=w1166) -> (element=w1165:refnum<vi>)  [unwired: 1 in]
      n323 = case shown="거짓" w1168 {
        tunnel: w1167 -> [w1176 w1188]
        tunnel: [w1173 w1184] -> w1169
        tunnel: w1163 -> [w1174 w1186]
        tunnel: w1165 -> [w1175 w1182]
        tunnel: w1170 -> [w1172 w1180]
        tunnel: w1171 -> [_ w1183]
        tunnel: [w1174 w1179] -> w1164
        frame False {
          n324 = call-poly "Table Initialize.vi"("행의 개수"=w1172, "Table Ref"=w1175, "에러 입력"=w1176) -> ("에러 출력"=w1173:errorcluster)  [unwired: 6 in, 2 out]
        }
        frame True {
          n325 = call "Variables Data IO.vi"("Select"=Cmd_Var_Data_IO."Result", "error in"=w1188, "Func_ext"=w1186) -> ("error out"=w1178:errorcluster, "Data Out"=w1177:string[][], "Func_ext Out"=w1179:string)  [unwired: 6 in]
          n326 = call-poly "Table Initialize.vi"("행의 개수"=w1180, "Table Ref"=w1182, "Value"=w1177, "에러 입력"=w1178) -> ("에러 출력"=w1181:errorcluster)  [unwired: 5 in, 2 out]
          n327 = call "Enq Msg.vi"("에러 입력(에러 없음)"=w1181, "메세지"="Value Change", "큐 입력"=w1183) -> ("에러 출력"=w1184:errorcluster)  [unwired: 7 in, 1 out]
        }
      }
    }
  }
  "에러 출력" <- w6
  "Func_ext Out" <- w14
